vi "Oxford-1820-Main.vi"() -> ()   [LabVIEW 2016]
uses:
  <instrlib>/Mercury iXX/Public/Controls/Unit String.ctl
  <instrlib>/Mercury iXX/Public/Libraries/Heater/Controls/Heater Device (Read).ctl
  <instrlib>/Mercury iXX/Public/Controls/Manufacturing Data.ctl
  <instrlib>/Mercury iXX/Public/Libraries/Heater/Controls/Heater Signals Cluster.ctl
  <instrlib>/Mercury iXX/Public/Libraries/Level Meter/Controls/Level Meter (Read).ctl
  <instrlib>/Mercury iXX/Public/Libraries/Level Meter/Controls/Nitrogen Configuration.ctl
  <instrlib>/Mercury iXX/Public/Libraries/Level Meter/Controls/Frequency Configuration.ctl
  <instrlib>/Mercury iXX/Public/Libraries/Level Meter/Controls/Signals.ctl
  <instrlib>/Mercury iXX/Public/Libraries/Level Meter/Controls/Helium Configuration.ctl
  <instrlib>/Mercury iXX/Public/Libraries/Level Meter/Controls/Resistance Configuration.ctl
  <instrlib>/Mercury iXX/Public/Libraries/Level Meter/Controls/Pre-Pulse.ctl
  <instrlib>/Mercury iXX/Public/Libraries/Level Meter/Controls/Pulse.ctl
  <instrlib>/Mercury iXX/Public/Libraries/Auxiliary/Controls/AUX Device (Read).ctl
  <instrlib>/Mercury iXX/Public/Libraries/Auxiliary/Controls/AUX Signals (Read).ctl
  <instrlib>/Mercury iXX/Public/Libraries/Magnet/Controls/Device (Read).ctl
  <instrlib>/Mercury iXX/Public/Libraries/Magnet/Controls/Signals (Read).ctl
  <instrlib>/Mercury iXX/Public/Libraries/Magnet/Controls/Identifier.ctl
  <instrlib>/Mercury iXX/Public/Libraries/Temperature/Controls/Calibration Cluster.ctl
  <instrlib>/Mercury iXX/Public/Libraries/Temperature/Controls/Calibration Interpolation.ctl
  <instrlib>/Mercury iXX/Public/Libraries/Temperature/Controls/Excitation Cluster.ctl
  <instrlib>/Mercury iXX/Public/Libraries/Temperature/Controls/Excitation Type.ctl
  <instrlib>/Mercury iXX/Public/Libraries/Pressure/Controls/Pressure Signals Cluster.ctl
  <instrlib>/Mercury iXX/Public/Controls/Mercury Reference.ctl
  <instrlib>/Mercury iXX/Public/Controls/Comms Transport Layer.ctl
  <instrlib>/Mercury iXX/Private/Controls/Query Dynamic Reference.ctl
  Mercury - Typedefs/Status.ctl
  <instrlib>/Mercury iXX/Public/Libraries/Magnet/Controls/PSU Actions.ctl
  Mercury - Typedefs/Actions.ctl
  <instrlib>/Mercury iXX/Public/Libraries/Magnet/Controls/Switch Heater.ctl
  <instrlib>/Mercury iXX/Public/Controls/ISOBus Address.ctl
  <instrlib>/Mercury iXX/Public/Controls/Response String.ctl
  <userlib>/_OpenG.lib/error/error.llb/Filter Error Codes (Array)__ogtk.vi
  <instrlib>/Mercury iXX/Public/Libraries/System/Open/Open System.vi
  <instrlib>/Mercury iXX/Public/Libraries/System/Read/Catalogue (Read).vi
  <instrlib>/Mercury iXX/Public/Libraries/System/Read/Display Automatic Dimming (Read).vi
  <instrlib>/Mercury iXX/Public/Libraries/System/Read/Display Automatic Dimming Time (Read).vi
  <instrlib>/Mercury iXX/Public/Libraries/System/Read/Display Brightness (Read).vi
  <instrlib>/Mercury iXX/Public/Libraries/System/Read/Date (Read).vi
  <instrlib>/Mercury iXX/Public/Libraries/System/Read/Time (Read).vi
  <instrlib>/Mercury iXX/Public/Libraries/System/Read/DateTime (Read).vi
  <instrlib>/Mercury iXX/Public/Libraries/System/Read/HVer (Read).vi
  <instrlib>/Mercury iXX/Public/Libraries/System/Read/FVer (Read).vi
  <instrlib>/Mercury iXX/Public/Libraries/System/Read/Serial Number (Read).vi
  <instrlib>/Mercury iXX/Public/Libraries/System/Read/Flash Space (Read).vi
  <instrlib>/Mercury iXX/Public/Libraries/System/Read/Mode (Read).vi
  <instrlib>/Mercury iXX/Public/Libraries/System/Set/DateTime (Set).vi
  <instrlib>/Mercury iXX/Public/Libraries/Temperature/Open/Open Temperature Device.vi
  <instrlib>/Mercury iXX/Public/Libraries/Temperature/Configuration/Read/Serial Number (Read).vi
  <instrlib>/Mercury iXX/Public/Libraries/Temperature/Configuration/Read/Nickname (Read).vi
  <instrlib>/Mercury iXX/Public/Libraries/Temperature/Configuration/Read/Excitation Magnitude (Read).vi
  <instrlib>/Mercury iXX/Public/Libraries/Temperature/Configuration/Read/Temperature Sensor (Read).vi
  <instrlib>/Mercury iXX/Public/Libraries/Temperature/Configuration/Read/Excitation Type (Read).vi
  <instrlib>/Mercury iXX/Public/Libraries/Temperature/Configuration/Read/Calibration Hot Limit (Read).vi
  <instrlib>/Mercury iXX/Public/Libraries/Temperature/Configuration/Read/Calibration Cold Limit (Read).vi
  <instrlib>/Mercury iXX/Public/Libraries/Temperature/Signals/Read/Voltage (Read).vi
  <instrlib>/Mercury iXX/Public/Libraries/Temperature/Signals/Read/Temperature (Read).vi
  <instrlib>/Mercury iXX/Public/Libraries/Temperature/Configuration/Read/Temperature Device (Read).vi
  <instrlib>/Mercury iXX/Public/Libraries/Heater/Open/Open Heater Device.vi
  <instrlib>/Mercury iXX/Public/Libraries/Heater/Configuration/Read/Heater Device (Read).vi
  <instrlib>/Mercury iXX/Public/Libraries/Heater/Configuration/Read/Nickname (Read).vi
  <instrlib>/Mercury iXX/Public/Libraries/Heater/Configuration/Read/Serial Number (Read).vi
  <instrlib>/Mercury iXX/Public/Libraries/Heater/Configuration/Read/Voltage Limit (Read).vi
  <instrlib>/Mercury iXX/Public/Libraries/Heater/Configuration/Read/Nominal Resistance (Read).vi
  <instrlib>/Mercury iXX/Public/Libraries/Heater/Configuration/Read/Maximum Power (Read).vi
  <instrlib>/Mercury iXX/Public/Libraries/Heater/Signals/Read/Voltage (Read).vi
  <instrlib>/Mercury iXX/Public/Libraries/Heater/Signals/Read/Power (Read).vi
  <instrlib>/Mercury iXX/Public/Libraries/Heater/Signals/Read/Current (Read).vi
  <instrlib>/Mercury iXX/Public/Libraries/Auxiliary/Open/Open Auxiliary Device.vi
  <instrlib>/Mercury iXX/Public/Libraries/Auxiliary/Configuration/Read/Aux Device (Read).vi
  <instrlib>/Mercury iXX/Public/Libraries/Auxiliary/Configuration/Read/Serial Number (Read).vi
  <instrlib>/Mercury iXX/Public/Libraries/Auxiliary/Configuration/Read/Minimum Gas Flow (Read).vi
  <instrlib>/Mercury iXX/Public/Libraries/Auxiliary/Configuration/Read/Gas Flow Scaling (Read).vi
  <instrlib>/Mercury iXX/Public/Libraries/Auxiliary/Configuration/Read/Temperature Error Sensitivity (Read).vi
  <instrlib>/Mercury iXX/Public/Libraries/Auxiliary/Configuration/Read/Temperature Error Voltage Sensitivity (Read).vi
  <instrlib>/Mercury iXX/Public/Libraries/Auxiliary/Configuration/Read/Valve Gearing (Read).vi
  <instrlib>/Mercury iXX/Public/Libraries/Auxiliary/Configuration/Read/Stepper Speed (Read).vi
  <instrlib>/Mercury iXX/Public/Libraries/Auxiliary/Signals/Read/Position (Read).vi
  <instrlib>/Mercury iXX/Public/Libraries/Auxiliary/Signals/Read/Percent Open (Read).vi
  <instrlib>/Mercury iXX/Public/Libraries/Pressure/Open/Open Pressure Device.vi
  <instrlib>/Mercury iXX/Public/Libraries/Pressure/Configuration/Read/Pressure Device (Read).vi
  <instrlib>/Mercury iXX/Public/Libraries/Pressure/Configuration/Read/Nickname (Read).vi
  <instrlib>/Mercury iXX/Public/Libraries/Pressure/Signals/Read/Current (Read).vi
  <instrlib>/Mercury iXX/Public/Libraries/Pressure/Signals/Read/Voltage (Read).vi
  <instrlib>/Mercury iXX/Public/Libraries/Level Meter/Open/Open Level Meter Device.vi
  <instrlib>/Mercury iXX/Public/Libraries/Level Meter/Configuration/Read/Level Meter Device (Read).vi
  <instrlib>/Mercury iXX/Public/Libraries/Level Meter/Configuration/Read/Serial Number (Read).vi
  <instrlib>/Mercury iXX/Public/Libraries/Level Meter/Configuration/Read/Helium Probe Resistance (Read).vi
  <instrlib>/Mercury iXX/Public/Libraries/Level Meter/Configuration/Read/Helium Pulse Mag (Read).vi
  <instrlib>/Mercury iXX/Public/Libraries/Level Meter/Configuration/Read/Helium Pulse Duration (Read).vi
  <instrlib>/Mercury iXX/Public/Libraries/Level Meter/Configuration/Read/Nitrogen Freq at 100 (Read).vi
  <instrlib>/Mercury iXX/Public/Libraries/Level Meter/Configuration/Read/Nitrogen Pulse Count Period (Read).vi
  <instrlib>/Mercury iXX/Public/Libraries/Level Meter/Signals/Read/Probe Resistance Helium (Read).vi
  <instrlib>/Mercury iXX/Public/Libraries/Level Meter/Signals/Read/Probe Level Helium (Read).vi
  <instrlib>/Mercury iXX/Public/Libraries/Level Meter/Signals/Read/Probe Count Nitrogen (Read).vi
  <instrlib>/Mercury iXX/Public/Libraries/Level Meter/Signals/Read/Probe Level Nitrogen (Read).vi
  <instrlib>/Mercury iXX/Public/Libraries/Magnet/Open/Open Magnet Device.vi
  <instrlib>/Mercury iXX/Public/Libraries/Magnet/Configuration/Read/Magnet Device (Read).vi
  <instrlib>/Mercury iXX/Public/Libraries/Magnet/Configuration/Read/Serial Number (Read).vi
  <instrlib>/Mercury iXX/Public/Libraries/Magnet/Configuration/Read/Bipolar Output (Read).vi
  <instrlib>/Mercury iXX/Public/Libraries/Magnet/Configuration/Read/Output Configuration (Read).vi
  <instrlib>/Mercury iXX/Public/Libraries/Magnet/Configuration/Read/Current Limit (Read).vi
  <instrlib>/Mercury iXX/Public/Libraries/Magnet/Configuration/Read/Current to Field Factor (Read).vi
  <instrlib>/Mercury iXX/Public/Libraries/Magnet/Configuration/Read/Switch Present (Read).vi
  <instrlib>/Mercury iXX/Public/Libraries/Magnet/Configuration/Read/Software Voltage Limit (Read).vi
  <instrlib>/Mercury iXX/Public/Libraries/Magnet/Signals/Read/Current Rate (Read).vi
  <instrlib>/Mercury iXX/Public/Libraries/Magnet/Configuration/Read/PSU Action Status (Read).vi
  <instrlib>/Mercury iXX/Public/Libraries/Temperature/Signals/Read/Resistance (Read).vi
  <instrlib>/Mercury iXX/Public/Libraries/Temperature/Configuration/Set/Excitation Magnitude (Set).vi
  <instrlib>/Mercury iXX/Public/Libraries/Magnet/Signals/Read/Switch Heater Status (Read).vi
  <instrlib>/Mercury iXX/Public/Libraries/Magnet/Signals/Read/Current (Read).vi
  <instrlib>/Mercury iXX/Public/Libraries/Magnet/Signals/Read/Voltage (Read).vi
  <instrlib>/Mercury iXX/Public/Libraries/Magnet/Signals/Read/Field (Read).vi
  <instrlib>/Mercury iXX/Public/Libraries/Magnet/Signals/Read/Target Field Rate (Read).vi
  <instrlib>/Mercury iXX/Public/Libraries/Magnet/Signals/Read/Target Field (Read).vi
  <instrlib>/Mercury iXX/Public/Libraries/Magnet/Signals/Read/Persistant Field (Read).vi
  <instrlib>/Mercury iXX/Public/Libraries/Magnet/Configuration/Set/PSU Action Status (Set).vi
  <instrlib>/Mercury iXX/Public/Libraries/Magnet/Signals/Read/Persistant Current (Read).vi
  <instrlib>/Mercury iXX/Public/Libraries/Magnet/Signals/Set/Switch Heater No Check (Set).vi
  <instrlib>/Mercury iXX/Public/Libraries/Magnet/Signals/Set/Target Field Rate (Set).vi
  <instrlib>/Mercury iXX/Public/Libraries/Magnet/Signals/Set/Target Field (Set).vi
  <instrlib>/Mercury iXX/Public/Libraries/Lambda/Open/Open Lambda Device.vi
  <instrlib>/Mercury iXX/Public/Libraries/Lambda/Configuration/Set/Lambda Flow Auto (Set).vi
  <instrlib>/Mercury iXX/Public/Libraries/Level Meter/Configuration/Set/Pulse Slow-Fast (Set).vi
  <instrlib>/Mercury iXX/Public/Libraries/Lambda/Configuration/Set/Lambda Percentage Flow (Set).vi
  <instrlib>/Mercury iXX/Mercury iXX.lvlib
  <instrlib>/Mercury iXX/Public/Libraries/Pressure.lvlib
  <instrlib>/Mercury iXX/Public/Libraries/System.lvlib
  <instrlib>/Mercury iXX/Public/Libraries/Temperature.lvlib
  <instrlib>/Mercury iXX/Public/Libraries/Auxiliary.lvlib
  <instrlib>/Mercury iXX/Public/Libraries/Magnet.lvlib
  <instrlib>/Mercury iXX/Public/Libraries/Level Meter.lvlib
  <instrlib>/Mercury iXX/Public/Libraries/Lambda.lvlib
  <instrlib>/Mercury iXX/Public/Libraries/System/Controls/User Mode.ctl
  <instrlib>/Mercury iXX/Public/Libraries/System/Set/Mode (Set).vi
  <instrlib>/Mercury iXX/Public/Libraries/Heater.lvlib
  <instrlib>/Mercury iXX/Public/Libraries/Magnet/Configuration/Set/Switch Heater Current (Set).vi
panel:
  out "LPF ON":timestamp
  in  "Tab Control":T1(tab)
  out "LEDs":bool[](array[boolean])
  out "Iteration Time":dbl
  in  "Percentage Open":dbl=100.0 format="%#_13g"
  out "PS Heat on or off (sec)":dbl format="%<%H:%M:%S>t"
  out "LPF on (min)":dbl=5373.0 format="%<%H:%M:%S>t"
  out "Magnet Status 2":string
  in  "OK":bool
  out "LPF Resistance":dbl=4.2075 format="%_3f ohms"
  out "Magnet Resistance":dbl=3.8705 format="%_3f ohms"
  out "ETA":timestamp format="%<%I:%M:%S %p\n%m/%d/%y>T"
  in  "Open Needle Valve":bool
  in  "Close Needle Valve":bool
  in  "Lambda":bool
  out "LPF Pressure":dbl format="%_5f mB"
  out "LPF Needle Valve (%)":dbl format="%_6g"
  out "LPF Temperature":dbl=4.2075 format="%_2f K"
  out "Magnet Temperature":dbl=3.8705 format="%_2f K"
  out "He LVL Chart":dbl(slide)=52.0833 scale=0.0..100.0
  out "N2 LVL Chart":dbl(slide)=61.3025 scale=0.0..100.0
  in  "Remote Mode":bool
  out "Power Supply Field (T)":dbl=0.0001 format="%#.5f"
  out "Magnet Field (T)":dbl format="%.5f"
  out "Voltage (V)":dbl=-0.0003 format="%.5f"
  out "Current (A)":dbl=0.0006 format="%.5f"
  out "N2 LEVEL":dbl=61.3025 format="%.0f %"
  out "He LEVEL":dbl=52.0833 format="%.0f %"
  in  "Fast/Slow Fill":bool
  out "Magnet Field (T)":dbl(knob) caption="Voltage (V)" scale=-20.0..20.0
  out "SWITCH HEATER":bool
  in  "PS Heat":bool
  in  "Clamp":bool
  in  "To Set":bool
  in  "To Zero":bool
  in  "Hold":bool
  out "Magnet Status":string="Clamped"
  out "Target Field Rate (T/min)":dbl=1.0 format="%.5f"
  out "Target Field (T)":dbl format="%#.5f"
  in  "Target Rate (T/min)":dbl=0.1 format="%.5f"
  in  "Target Field (T)":dbl format="%#.5f"
  in  "Send to IPS":bool
  out "Voltage (V)":dbl(knob)=-0.0003 scale=-10.0..10.0
  out "Current (A)":dbl(knob)=0.0006 scale=-180.0..180.0
  in  "Mercury Functions":T2(tab)=enum."ITC: Temperature"
  out "time stamp":timestamp=timestamp(3543841780 s since 1904-01-01)
  out "Free Space":i32=166384 caption="Free Space (KB)"
  out "Set Date Response":string="VALID"
  out "String":string="NORM" caption="User Mode"
  out "Date":string="2016:04:18"
  out "Time":string="11:29:40"
  out "Hardware Version":string="65"
  out "Firmware Version":string="2.2.6.20"
  out "Serial Number":string="154650110"
  out "ITC Devices":string[](array[string])=["DB4.G1:AUX", "DB8.P1:PRES", "MB0.H1:HTR", "MB1.T1:TEMP"]
  out "S/W Version(s)":string[](array[string])=["2.2.6.20\n"]
  out "Serial Number(s)":string[](array[string])=["154650110"]
  out "# of Instruments":i32=1
  out "Automatic Dimming":string="OFF"
  out "Dimming Time":string="5"
  out "Display Brightness":string="100"
  in  "ITC IP Address":string="130.49.180.101"
  out "Excitation Magnitude":dbl=5.0
  out "Sensor Type":string="NTC"
  out "Excitation Type":string="UNIP"
  out "Hot Limit":dbl=1000.0
  out "H Unit":T3="K"
  out "Cold Limit":dbl=1000.0
  out "C Unit":T3="K"
  out "Unit":T3
  out "Voltage":dbl=0.005
  out "V Unit":T3="V"
  out "Temperature":dbl=4.2075
  out "T Unit":T3="K"
  out "Temp S/N":string="154650110"
  out "T Nickname":string="Mag_AB_MB1"
  out "ITC Calibration":T4
  out "ITC Excitation":T6
  out "ITC Manufacturing":T8
  out "Heater Device Settings":T9={"Manufacturing"={"Hardware Version"="65", "Firmware Version"="2.3", "Serial Number"="154650110"}, "Nickname"="MB0.H1", "Voltage Limit"="1", "Nominal Resistance"="10", "Maximum Power"="0.1000", "Heater Signals"={"Voltage"="0.0507V", "Current"="-0.0000A", "Power"="0.0000W"}, "Status"="2"}
  out "Htr C Unit":T3="A"
  out "Htr P Unit":T3="W"
  out "Htr V Unit":T3="V"
  out "Htr Current":dbl=-0.0
  out "Htr Power":dbl
  out "Htr Voltage":dbl=0.0507
  out "Power Unit":T3
  out "Volt Unit":T3
  out "Res Unit":T3
  out "Maximum Power":dbl=0.1
  out "Htr Resistance":dbl=10.0
  out "Htr Voltage Limit":dbl=1.0
  out "Htr S/N":string="154650110"
  out "Htr Nickname":string="MB0.H1"
  out "Nickname":string="Lam_P_DB8"
  out "Current":dbl=-0.0
  out "Voltage":dbl=-8.219999999999999e-05
  out "Manufacturing":T8
  out "Pressure Signals":T11
  out "Auxiliary Device Details":T12={"Manufacturing"={"Hardware Version"="65", "Firmware Version"="3.1", "Serial Number"="154650084"}, "Min Flow"=0.0, "Scaling Factor"=50.0, "Temp Err"=9.0, "Temp V Err"=11.0, "Gear"=2, "Speed"=2, "Signals"={"Position"=0.0, "% Open"=0.0, "I0"="ON", "I1"="OFF", "I2"="OFF", "I3"="OFF", "O0"="OFF", "O1"="OFF", "O2"="OFF", "O3"="OFF"}, "Nickname"="DB4.G1", "Status"="0"} {"Signals"."% Open" min=0.0 max=100.0 step=0.1 format="%.4f"; "Signals"."Position" max=20.0 step=1.0 format="%.4f"; "Speed" max=7 step=1; "Gear" max=7 step=1; "Temp V Err" min=0.0 max=20.0 step=0.1; "Temp Err" min=0.0 max=20.0 step=0.1; "Scaling Factor" min=0.0 max=99.0 step=0.1; "Min Flow" min=0.0 max=20.0 step=0.1}
  out "Aux S/N":string="154650084"
  out "Min Flow":dbl caption="Minimum Gas Flow" format="%#.1f"
  out "Scaling Factor":dbl=50.0 caption="Gas Flow Scaling Factor" format="%#.1f"
  out "Temp Err":dbl=9.0 caption="Temperature Error Sensitivity" format="%#.1f"
  out "Temp V Err":dbl=11.0 caption="Temperature Voltage Error Sensitivity" format="%#.1f"
  out "Gear":u32=2 caption="Valve Gearing"
  out "Speed":u32=2 caption="Stepper Speed"
  out "Unit 2":T3
  out "Unit 3":T3
  out "Unit 4":T3
  out "Unit 5":T3
  out "Unit 6":T3
  out "Unit 7":T3
  out "Position":u32
  out "% Open":dbl caption="Percentage Open (%)"
  out "Unit":T3
  out "Unit":T3="%"
  out "time stamp 2":timestamp=timestamp(3543841781 s since 1904-01-01)
  out "Free Space 2":i32=166316 caption="Free Space (KB)"
  out "Set Date Response 2":string="VALID"
  out "String 2":string="NORM" caption="User Mode"
  out "Date 2":string="2016:04:18"
  out "Time 2":string="11:29:45"
  out "Hardware Version 2":string="65"
  out "Firmware Version 2":string="2.2.6.20"
  out "Serial Number 2":string="153350063"
  out "IPS Devices":string[](array[string])=["DB3.L1:LVL", "GRPX:PSU", "GRPY:PSU", "GRPZ:PSU", "MB1.T1:TEMP", "PSU.M1:PSU", "PSU.M2:PSU", "PSU.M3:PSU"]
  out "S/W Version(s) 2":string[](array[string])=["2.2.6.20\n"]
  out "Serial Number(s) 2":string[](array[string])=["153350063"]
  out "# of Instruments 2":i32=1
  out "Automatic Dimming 2":string="OFF"
  out "Dimming Time 2":string="5"
  out "Display Brightness 2":string="100"
  in  "IPS IP Address":string="130.49.180.102"
  out "LVL Device DetailSettings":T14={"Manufacturing"={"Hardware Version"="65", "Firmware Version"="2.2", "Serial Number"="152450013"}, "Nitrogen Configuration"={"Frequency Configuration"={"Freq 0%"=0.0, "Freq 100%"=0.0}, "Pulse Period"=0.0}, "Signals"={"Helium Signals"={"Resistance"=75.5626, "Level"=52.0833}, "Nitrogen Signals"={"Count"=8800.0, "Freq"=487361.0, "Level"=61.3445}}, "Nickname"="DB3.L1", "Status"="0", "Helium Configuration"={"Resistance Configuration"={"Res 0%"=0.0, "Res 100%"=0.0}, "Pre-Pulse"={"Magnitude"=0.0, "Duration"=0.0}, "Pulse"={"Magnitude"=0.0, "Duration"=0.0, "Delay"=0.0}}}
  out "LVL S/N":string="152450013"
  out "LVL P Magnitude":dbl=125.0 caption="Pulse Magnitude (mA)"
  out "LVL P Duration":dbl=5.0 caption="Pulse Duration (s)"
  out "N Freq 100%":dbl=7880.0 caption="Frequency at 100% (Hz)"
  out "N Pulse Period":dbl=1000.0 caption="Pulse Period (ms)"
  out "He Res Config":T19={"Res 0%"=149.0, "Res 100%"=8.0}
  out "He Resistance":dbl=75.5626 caption="Resistance (Ohms)"
  out "He Level":dbl=52.0833 caption="Helium Level (%)"
  out "N Counter":u32 caption="Counter"
  out "N Level":dbl=61.3445 caption="Nitrogen Level (%)"
  out "Excitation Magnitude 2":dbl=5.0
  out "Sensor Type 2":string="NTC"
  out "Excitation Type 2":string="UNIP"
  out "Hot Limit 2":dbl=1000.0
  out "H Unit 2":T3="K"
  out "Cold Limit 2":dbl=1000.0
  out "C Unit 2":T3="K"
  out "Unit 12":T3
  out "Voltage 2":dbl=0.005
  out "V Unit 2":T3="V"
  out "Temperature 2":dbl=3.8706
  out "T Unit 2":T3="K"
  out "Temp S/N 2":string="153350063"
  out "T Nickname 2":string="MB1.T1"
  out "IPS Calibration":T4
  out "IPS Excitation":T6
  out "IPS Manufacturing":T8
  out "Magnet Device Details":T22={"Manufacturing"={"Hardware Version"="NOT_FOUND", "Firmware Version"="NOT_FOUND", "Serial Number"="NOT_FOUND"}, "Nickname"="GRPZ", "Bipolar Output"="ON", "String"="PARA", "Current Limit"=174.0, "AtoB"=8.688, "Inductance"=39.406, "Switch Present"="PSU.M1", "Swh Htr Current"=86.0, "SW VLIM"=9.0, "V Trans Time"=1000.0, "Magnet PSU Signals"={"Voltage"=-0.0002, "Current"=0.0002, "Current Rate"=100.0, "Field"=0.0001, "Field Rate"=11.5101, "Persistant Current"=0.0003, "Persistant Field"=0.0, "Target Current"=0.0, "Target Field"=0.0, "Target Current Rate"=8.688, "Target Field Rate"=1.0, "Switch Heater Status (SWHT)"="OFF", "Switch Heater Status (SWHN)"="OFF"}, "PSU Action"="CLMP", "Status"="40000000", "Level Limit"=0.0, "Temperature Limit"=999.0} {"Temperature Limit" format="%#.1f"; "Level Limit" format="%#.1f"; "V Trans Time" format="%#.1f"; "SW VLIM" format="%#.1f"; "Swh Htr Current" format="%#.1f"; "Inductance" format="%#.1f"; "AtoB" format="%#.1f"; "Current Limit" format="%#.1f"}
  out "Mag S/N":string="NOT_FOUND"
  out "Bipolar Output":string="ON"
  out "Out Config":string="PARA" caption="Output Configuration"
  out "Current Limit":dbl=174.0 caption="Current Limit (A)" format="%#.1f"
  out "AtoB":dbl=8.688 caption="Current Field Factor (A/T)" format="%#.1f"
  out "Switch Present":string="PSU.M1"
  out "SW VLIM":dbl=9.0 caption="Software Voltage Limit (V)" format="%#.1f"
  out "Unit 8":T3
  out "Unit 9":T3
  out "Unit 10":T3
  out "Current Rate":dbl=100.0
  out "PSU Act Stat":string="CLMP" caption="PSU Action Status"
  out "Unit 11":T3="A/min"
  in  "Device Identifier":T24="GRPZ"
  out "M3 Voltage":dbl
  out "M3 Current":dbl
  out "M2 Voltage":dbl
  out "M2 Current":dbl
  out "M1 Voltage":dbl
  out "M1 Current":dbl
  out "Error List":T25(array[cluster])
  out "PS ON/OFF":timestamp format="%<%I:%M:%S %p>T"
  # "v2017/09/27"
  # "Voltage (V)"
  # "Magnet (T)"
  # "Current (A)"
  # "Slow Rates\nCurrent Range (A)     Field Range (T)    Rate (T/min)\n0       -- 100        0    -- 11.5       0.91\n100     -- 150        11.5 -- 17.2       0.23\n150     -- 155.467    17.2 -- 18         0.11\n155.567 -- 172.471    18   -- 20         0.11"
  # "Fast Rates\nCurrent Range (A)     Field Range (T)    Rate (T/min)\n0       -- 155.467    0    -- 18         1.0\n155.567 -- 172.471    18   -- 20         0.25"
  # "ITC: 101\nIPS: 102\nIPS VR: 67"
  # "ITC: 101\nIPS: 102\nIPS VR: 67"
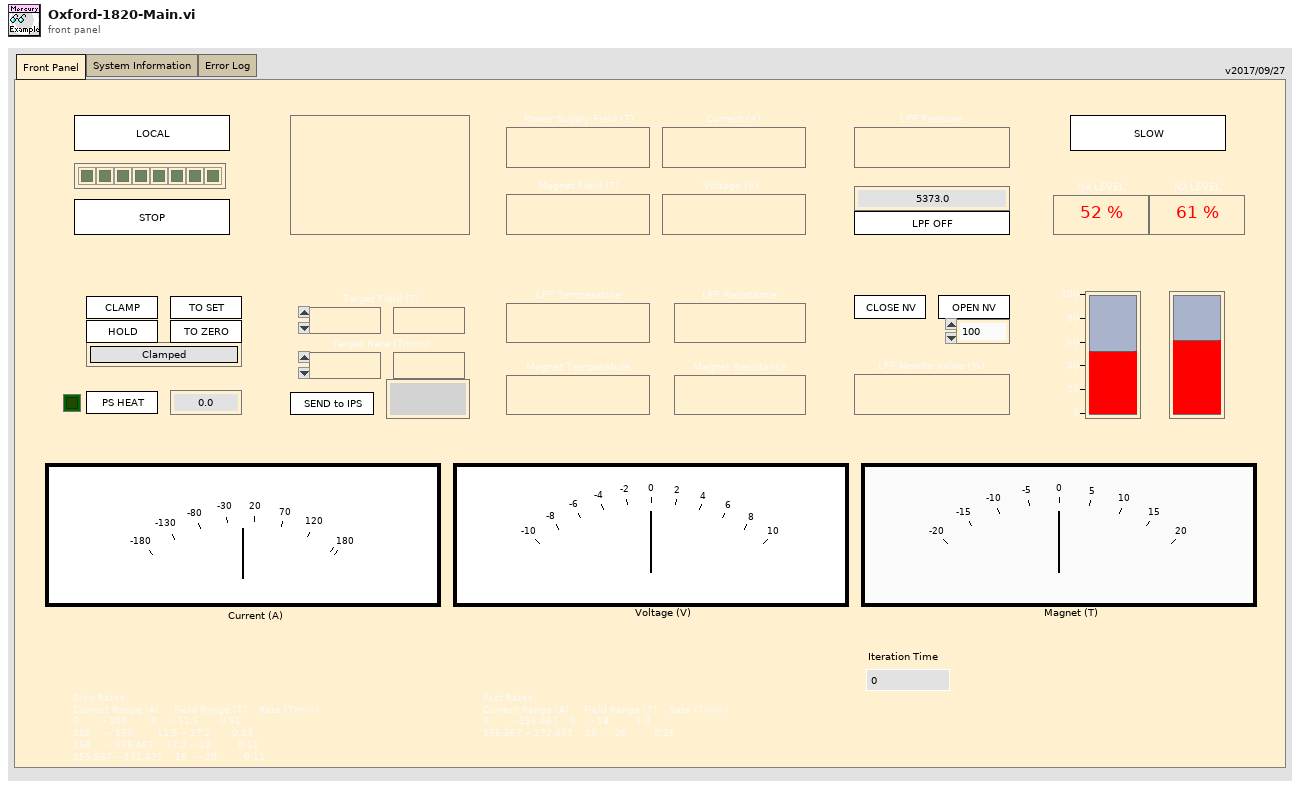
[diagram p1: front panel]
types:
  T1 = enum32{"Front Panel", "System Information", "Error Log"}
  T2 = enum32{"ITC: System", "ITC: Temperature", "ITC: Heater", "ITC: Pressure", "ITC: Auxiliary", "IPS: System", "IPS: Level Meter", "IPS: Temperature", "IPS: Magnet"}
  T3 = typedef "Mercury iXX.lvlib/Unit String.ctl" = string
  T4 = typedef "Mercury iXX.lvlib/Temperature.lvlib/Calibration Cluster.ctl" = cluster{"Filename":string, "Interpolation":T5, "Scaling Factor":string, "Offset Factor":string, "Hot Limit":string, "Cold Limit":string, "Last Calibration":string, "Reference":string}
  T5 = typedef "Mercury iXX.lvlib/Temperature.lvlib/Calibration Interpolation.ctl" = string
  T6 = typedef "Mercury iXX.lvlib/Temperature.lvlib/Excitation Cluster.ctl" = cluster{"Excitation Type":T7, "Magnitude":string}
  T7 = typedef "Mercury iXX.lvlib/Temperature.lvlib/Excitation Type.ctl" = string
  T8 = typedef "Mercury iXX.lvlib/Manufacturing Data.ctl" = cluster{"Hardware Version":string, "Firmware Version":string, "Serial Number":string}
  T9 = typedef "Mercury iXX.lvlib/Heater.lvlib/Heater Device (Read).ctl" = cluster{"Manufacturing":T8, "Nickname":string, "Voltage Limit":string, "Nominal Resistance":string, "Maximum Power":string, "Heater Signals":T10, "Status":string}
  T10 = typedef "Mercury iXX.lvlib/Heater.lvlib/Heater Signals Cluster.ctl" = cluster{"Voltage":string, "Current":string, "Power":string}
  T11 = typedef "Mercury iXX.lvlib/Pressure.lvlib/Pressure Signals Cluster.ctl" = cluster{"Voltage":string, "Current":string, "Power":string, "Pressure":string}
  T12 = typedef "Mercury iXX.lvlib/Auxiliary.lvlib/AUX Device (Read).ctl" = cluster{"Manufacturing":T8, "Min Flow":dbl, "Scaling Factor":dbl, "Temp Err":dbl, "Temp V Err":dbl, "Gear":u32, "Speed":u32, "Signals":T13, "Nickname":string, "Status":string}
  T13 = typedef "Mercury iXX.lvlib/Auxiliary.lvlib/AUX Signals (Read).ctl" = cluster{"Position":dbl, "% Open":dbl, "I0":string, "I1":string, "I2":string, "I3":string, "O0":string, "O1":string, "O2":string, "O3":string}
  T14 = typedef "Mercury iXX.lvlib/Level Meter.lvlib/Level Meter (Read).ctl" = cluster{"Manufacturing":T8, "Nitrogen Configuration":T15, "Signals":T17, "Nickname":string, "Status":string, "Helium Configuration":T18}
  T15 = typedef "Mercury iXX.lvlib/Level Meter.lvlib/Nitrogen Configuration.ctl" = cluster{"Frequency Configuration":T16, "Pulse Period":dbl}
  T16 = typedef "Mercury iXX.lvlib/Level Meter.lvlib/Frequency Configuration.ctl" = cluster{"Freq 0%":dbl, "Freq 100%":dbl}
  T17 = typedef "Mercury iXX.lvlib/Level Meter.lvlib/Signals.ctl" = cluster{"Helium Signals":cluster{"Resistance":dbl, "Level":dbl}, "Nitrogen Signals":cluster{"Count":dbl, "Freq":dbl, "Level":dbl}}
  T18 = typedef "Mercury iXX.lvlib/Level Meter.lvlib/Helium Configuration.ctl" = cluster{"Resistance Configuration":T19, "Pre-Pulse":T20, "Pulse":T21}
  T19 = typedef "Mercury iXX.lvlib/Level Meter.lvlib/Resistance Configuration.ctl" = cluster{"Res 0%":dbl, "Res 100%":dbl}
  T20 = typedef "Mercury iXX.lvlib/Level Meter.lvlib/Pre-Pulse.ctl" = cluster{"Magnitude":dbl, "Duration":dbl}
  T21 = typedef "Mercury iXX.lvlib/Level Meter.lvlib/Pulse.ctl" = cluster{"Magnitude":dbl, "Duration":dbl, "Delay":dbl}
  T22 = typedef "Mercury iXX.lvlib/Magnet.lvlib/Device (Read).ctl" = cluster{"Manufacturing":T8, "Nickname":string, "Bipolar Output":string, "String":string, "Current Limit":dbl, "AtoB":dbl, "Inductance":dbl, "Switch Present":string, "Swh Htr Current":dbl, "SW VLIM":dbl, "V Trans Time":dbl, "Magnet PSU Signals":T23, "PSU Action":string, "Status":string, "Level Limit":dbl, "Temperature Limit":dbl}
  T23 = typedef "Mercury iXX.lvlib/Magnet.lvlib/Signals (Read).ctl" = cluster{"Voltage":dbl, "Current":dbl, "Current Rate":dbl, "Field":dbl, "Field Rate":dbl, "Persistant Current":dbl, "Persistant Field":dbl, "Target Current":dbl, "Target Field":dbl, "Target Current Rate":dbl, "Target Field Rate":dbl, "Switch Heater Status (SWHT)":string, "Switch Heater Status (SWHN)":string}
  T24 = typedef "Mercury iXX.lvlib/Magnet.lvlib/Identifier.ctl" = string
  T25 = cluster{"time":timestamp, "code":i32, "source":string}[]
  T26 = enum32{"invalid app kind", "Development System", "Run Time System", "Student Edition", "Embedded LabVIEW", "Evaluation", "Custom"}
  T27 = cluster{"time":timestamp, "code":i32, "source":string}
  T28 = enum32{"Invalid", "Standard", "Closed", "Hidden", "Minimized", "Maximized"}
  T29 = typedef "Status.ctl" = cluster{"Magnet Field":dbl, "PS Field":dbl, "Target Field":dbl, "Target Field Rate":dbl, "Voltage":dbl, "Current":dbl, "Switch":bool, "Mercury State":string}
  T30 = cluster{"Magnet Field":dbl, "PS Field":dbl, "Target Field":dbl, "Target Field Rate":dbl, "Voltage":dbl, "Current":dbl}
  T31 = typedef "Actions.ctl" = cluster{"Hold":bool, "Clamp":bool, "To Set":bool, "To Zero":bool, "Send to IPS":bool, "PS Heat":bool, "Lambda":bool}
  T32 = typedef "Mercury iXX.lvlib/Magnet.lvlib/PSU Actions.ctl" = string
  T33 = typedef "Mercury iXX.lvlib/Magnet.lvlib/Switch Heater.ctl" = string
  T34 = typedef "Mercury iXX.lvlib/ISOBus Address.ctl" = i32
  T35 = typedef "Mercury iXX.lvlib/Response String.ctl" = string
  T36 = typedef "Mercury iXX.lvlib/Mercury Reference.ctl" = cluster{"Comms":refnum<visa-resource-name>, "Device ID":string[], "Comms Layer":T37, "Command":string, "Query reference":T38}
  T37 = typedef "Mercury iXX.lvlib/Comms Transport Layer.ctl" = enum16{"Ethernet TCP/IP", "USB", "ISOBus - RS-232", "GPIB"}
  T38 = typedef "Mercury iXX.lvlib/Query Dynamic Reference.ctl" = refnum<vi>
  T39 = cluster{"Core":cluster{"Current VI Reference":refnum<vi>, "Close Panel on Exit?":bool}, "Mercury ITC Ref":T36, "Mercury IPS Ref":T36, "sentinel":bool, "Error Log":cluster{"time":timestamp, "code":i32, "source":string}[], "read ITC T?":bool, "counter":i32}
  T40 = typedef "Filtered Error Details - Cluster__ogtk.ctl" = cluster{"code":i32, "source":string}
  T41 = cluster{"Current VI Reference":refnum<vi>, "Close Panel on Exit?":bool}
  T42 = typedef "Mercury iXX.lvlib/System.lvlib/User Mode.ctl" = string
  T43 = typedef "Mercury iXX.lvlib/Temperature.lvlib/Temperature Sensor Type.ctl" = string
  T44 = typedef "Mercury iXX.lvlib/Temperature.lvlib/Temperature Device (Read).ctl" = cluster{"Manufacturing":T8, "Temperature Sensor Type":T43, "Excitation":T6, "Calibration":T4, "Control Loop":T45, "Temperature Signals":T46, "Nickname":string, "Status":string}
  T45 = typedef "Mercury iXX.lvlib/Temperature.lvlib/Loop Cluster.ctl" = cluster{"Heater":string, "Auxiliary":string, "Heater Auto":string, "Percentage Heat":string, "Temperature Set Point":string, "PID Auto (from file)":string, "P Value":string, "I Value":string, "D Value":string, "Auto PID Table Filename":string, "Flow Auto":string, "Target Heater Table":string, "Sweep mode":string, "Sweep Table Filename":string, "Percentage Flow":string}
  T46 = typedef "Mercury iXX.lvlib/Temperature.lvlib/Temperature Signals Cluster.ctl" = cluster{"Voltage":string, "Current":string, "Power":string, "Resistance":string, "Temperature":string, "Sensitivity":string, "Reference":string}
  T47 = typedef "Mercury iXX.lvlib/Pressure.lvlib/Pressure Device (Read).ctl" = cluster{"Manufacturing":T8, "Temperature Sensor Type":T48, "Calibration":T49, "Control Loop":T51, "Pressure Signals":T11, "Nickname":string, "Status":string}
  T48 = typedef "Mercury iXX.lvlib/Pressure.lvlib/Pressure Sensor Type.ctl" = string
  T49 = typedef "Mercury iXX.lvlib/Pressure.lvlib/Calibration Cluster.ctl" = cluster{"Filename":string, "Interpolation":T50, "Scaling Factor":string, "Offset Factor":string, "High Limit":string, "Low Limit":string, "Last Calibration":string}
  T50 = typedef "Mercury iXX.lvlib/Pressure.lvlib/Calibration Interpolation.ctl" = string
  T51 = typedef "Mercury iXX.lvlib/Pressure.lvlib/Loop Cluster.ctl" = cluster{"Heater":string, "Auxiliary":string, "Heater Auto":string, "Percentage Heat":string, "Pressure Set Point":string, "PID Auto (from file)":string, "P Value":string, "I Value":string, "D Value":string, "Auto PID Table Filename":string, "Flow Auto":string, "Target Heater Table":string, "Sweep mode":string, "Sweep Table Filename":string, "Percentage Flow":string}
  T52 = typedef "Mercury iXX.lvlib/Magnet.lvlib/Output Configuration.ctl" = string
  T53 = typedef "Targets.ctl" = cluster{"Target Field (T)":dbl, "Target Field Rate (T/min)":dbl}
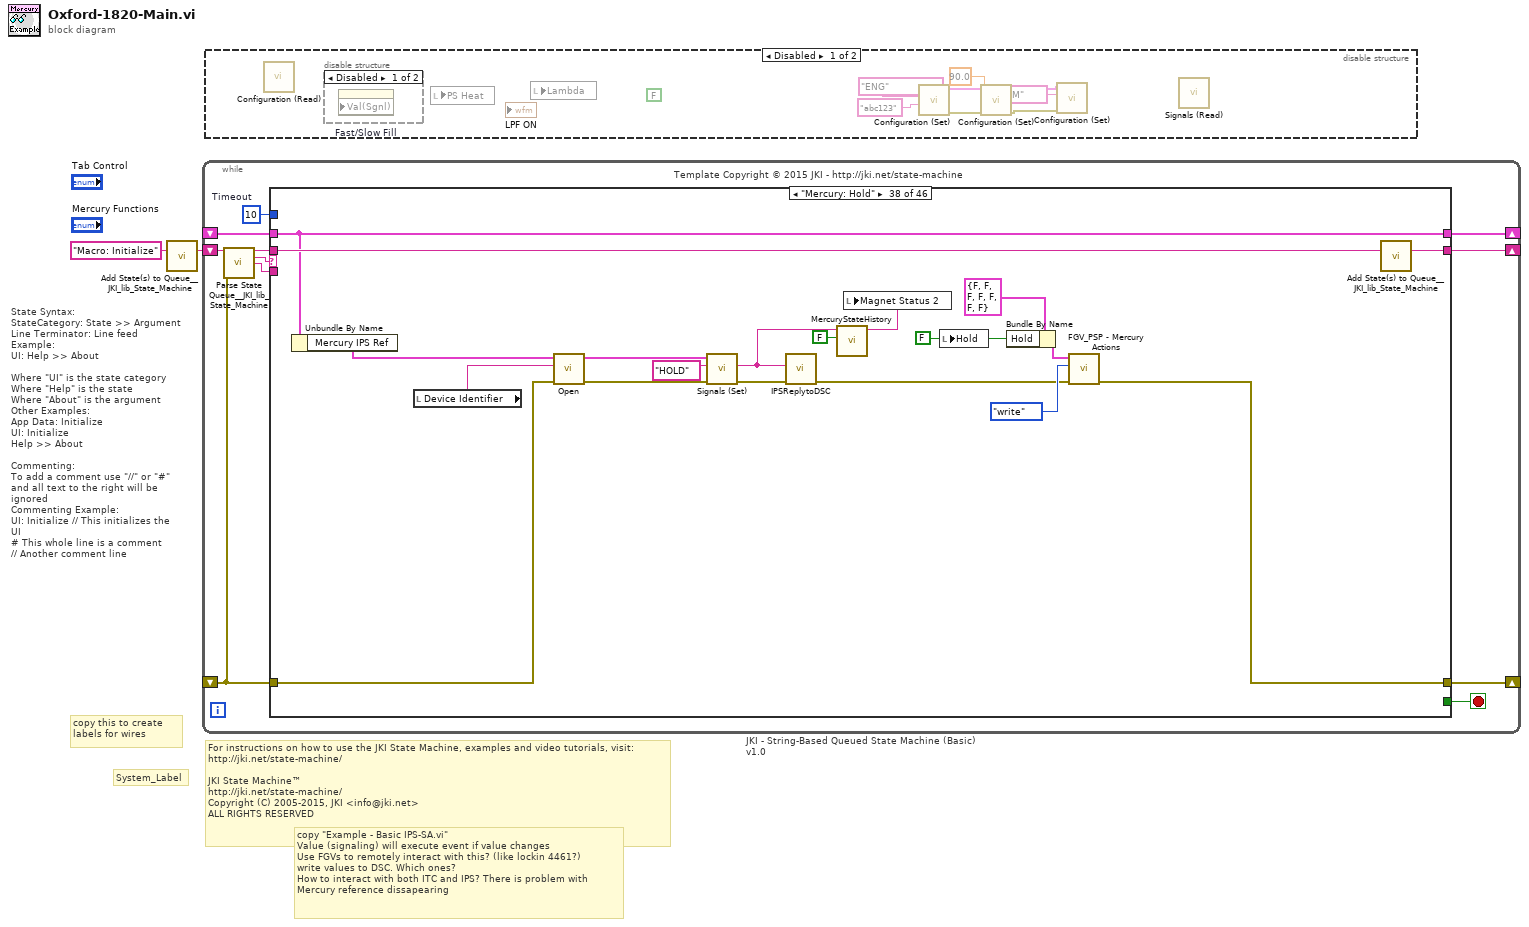
[diagram p0: block diagram]
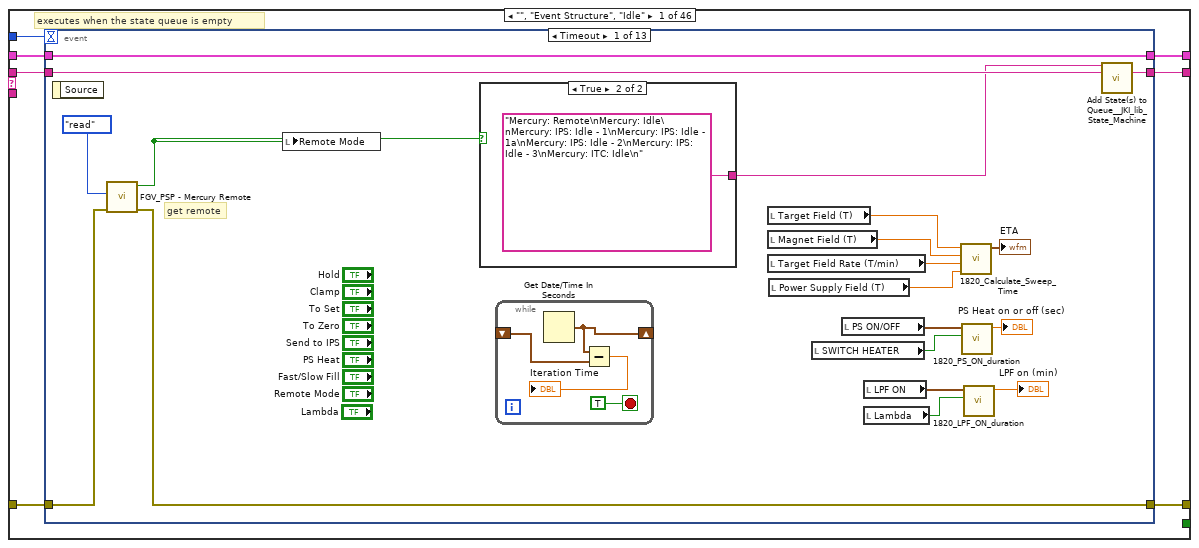
[diagram p4: hidden frame]
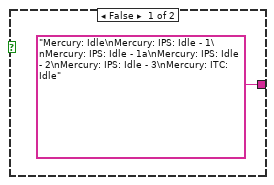
[diagram p5: hidden frame]
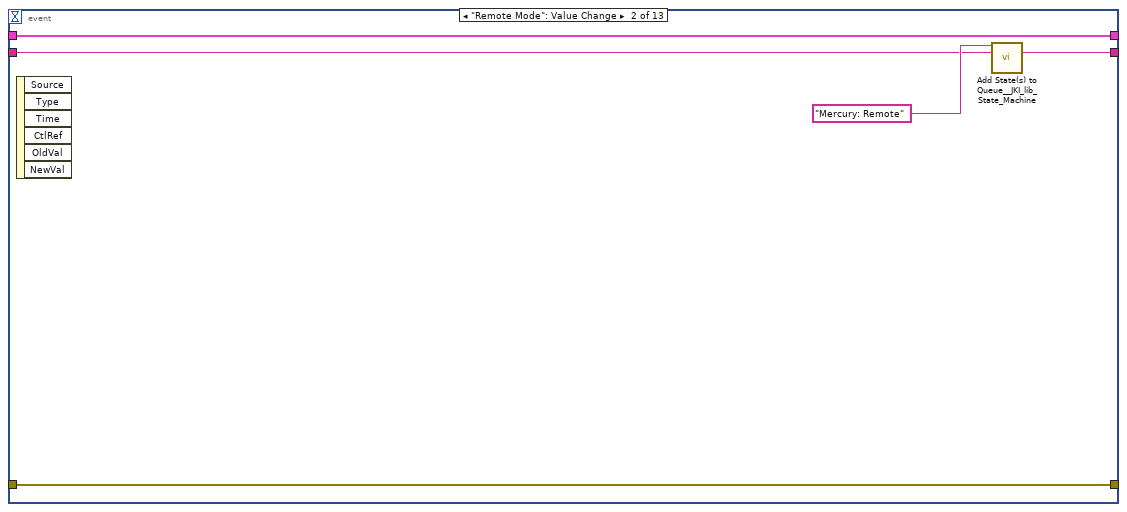
[diagram p6: hidden frame]
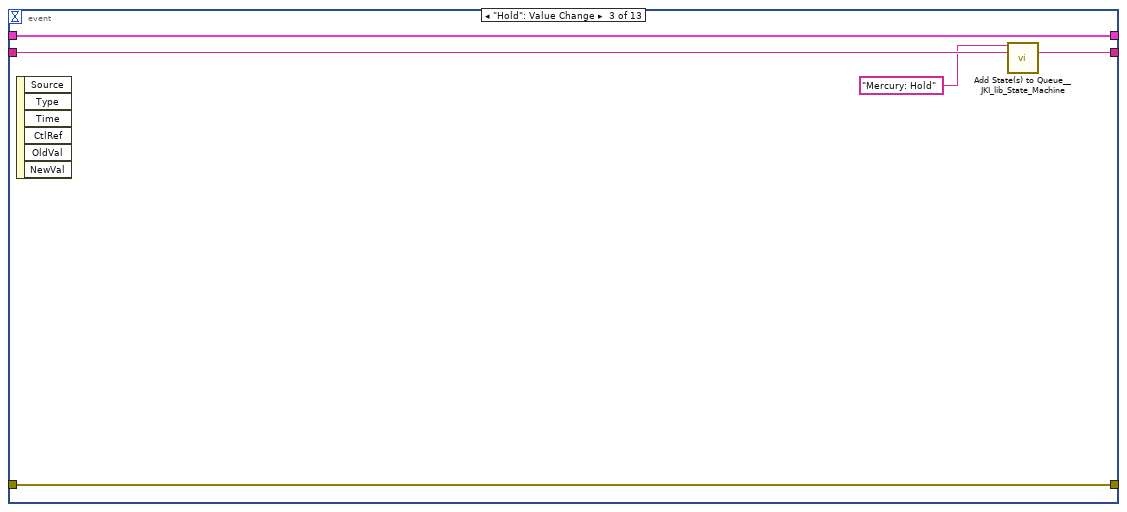
[diagram p7: hidden frame]
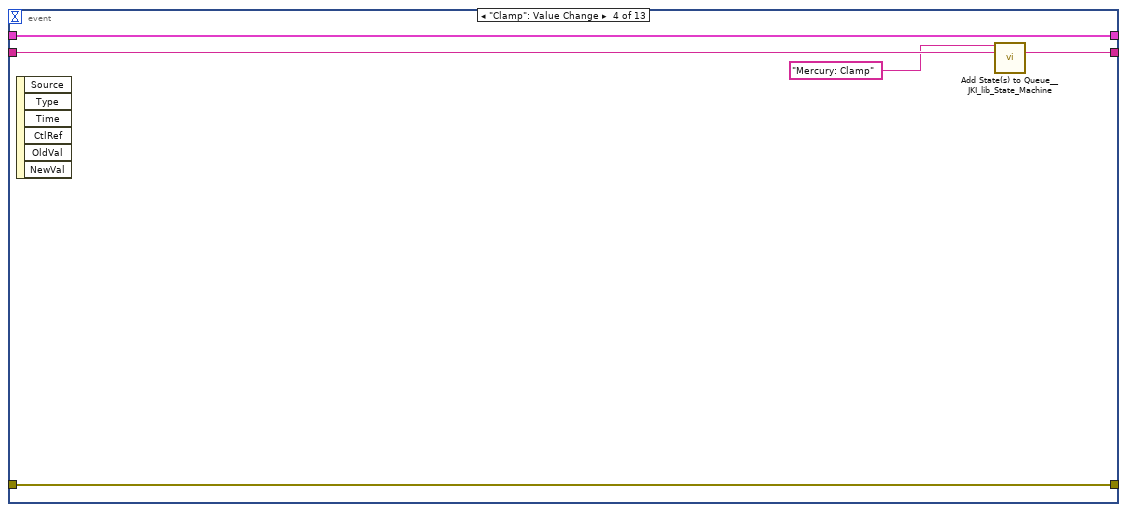
[diagram p8: hidden frame]
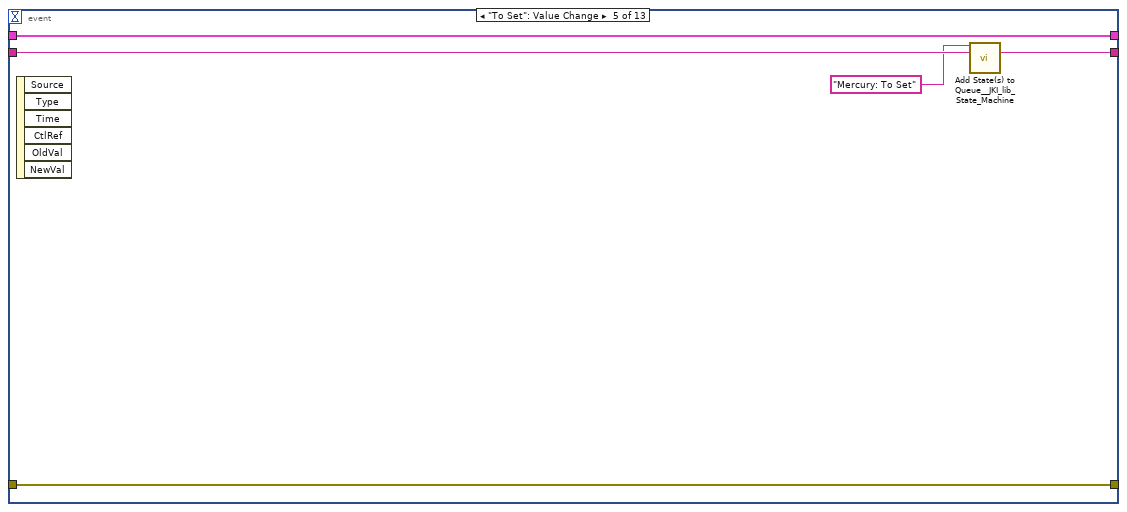
[diagram p9: hidden frame]
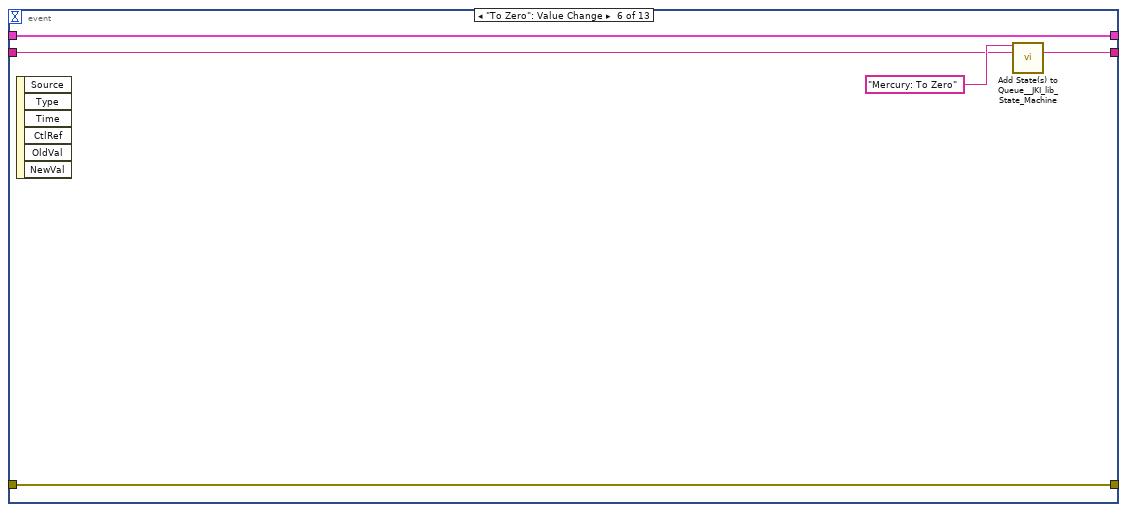
[diagram p10: hidden frame]
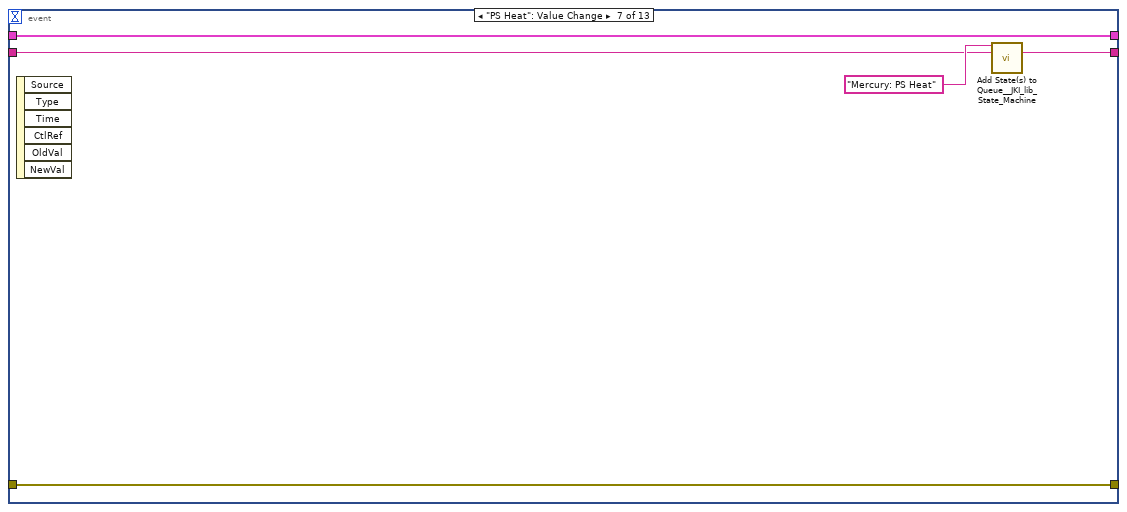
[diagram p11: hidden frame]
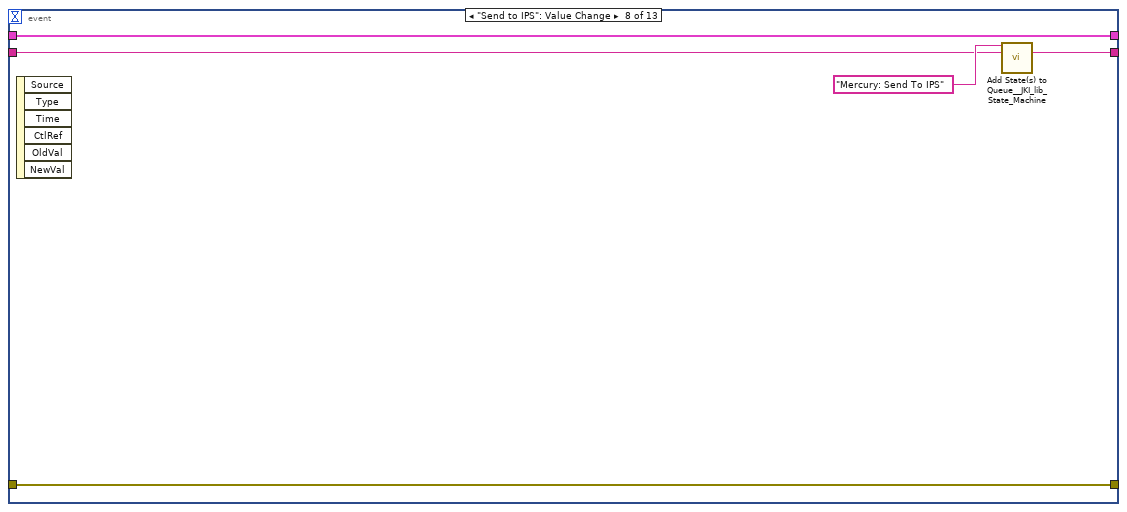
[diagram p12: hidden frame]
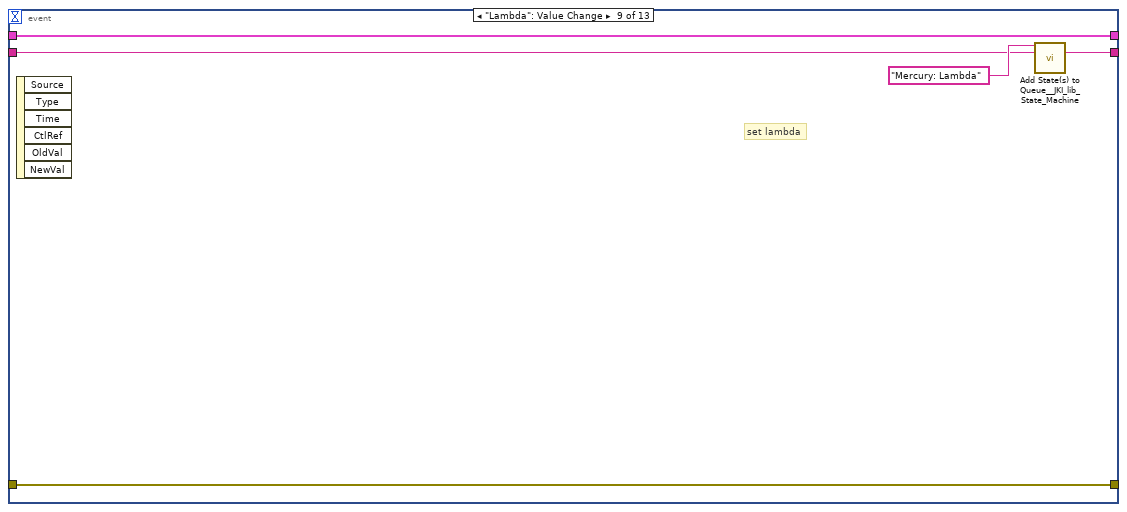
[diagram p13: hidden frame]
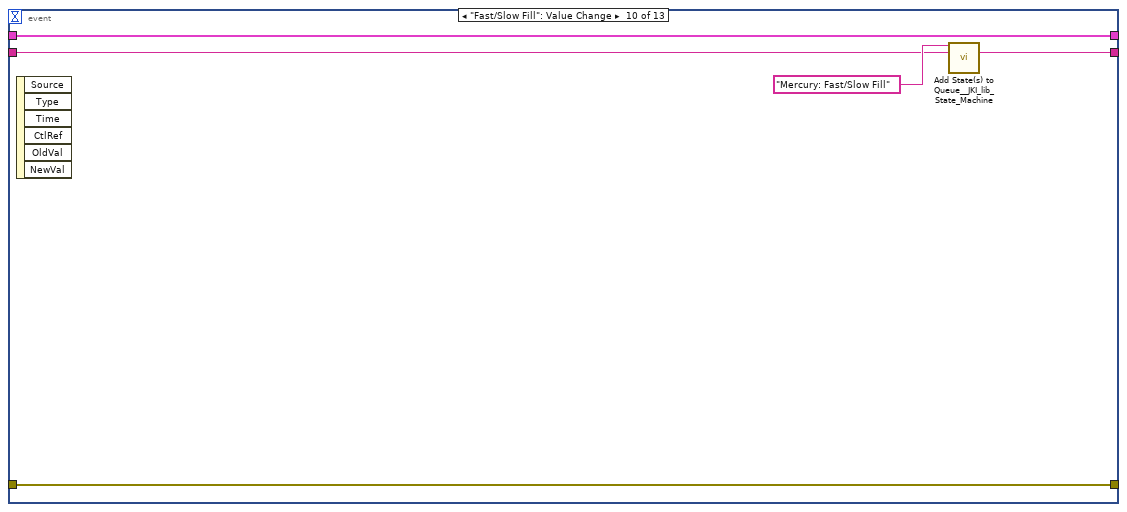
[diagram p14: hidden frame]
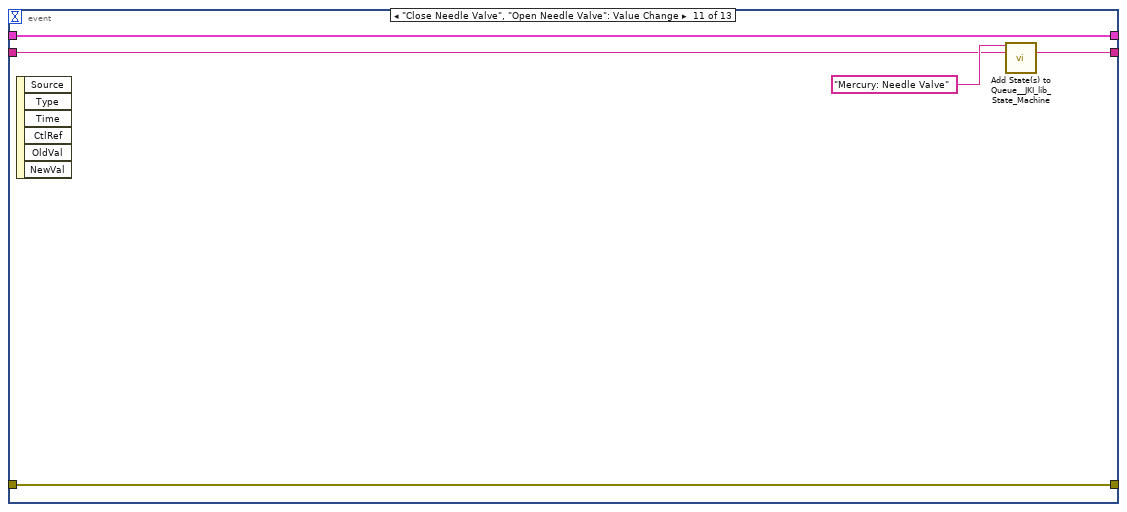
[diagram p15: hidden frame]
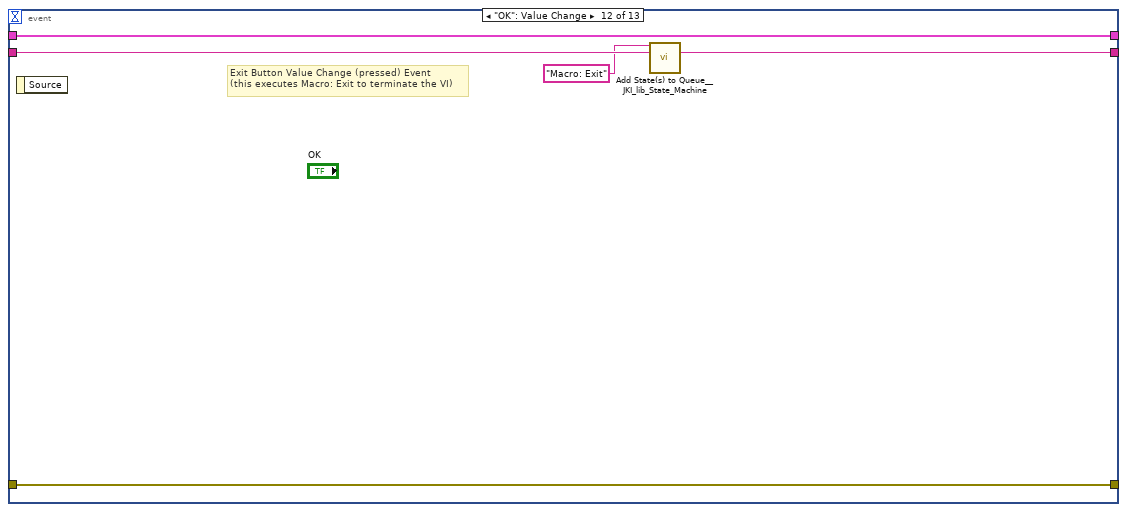
[diagram p16: hidden frame]
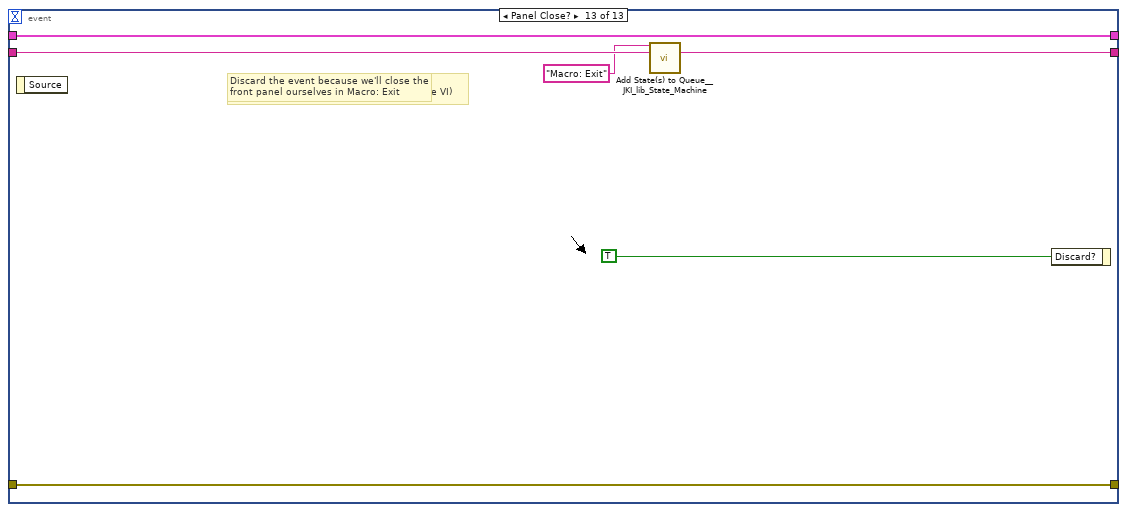
[diagram p17: hidden frame]
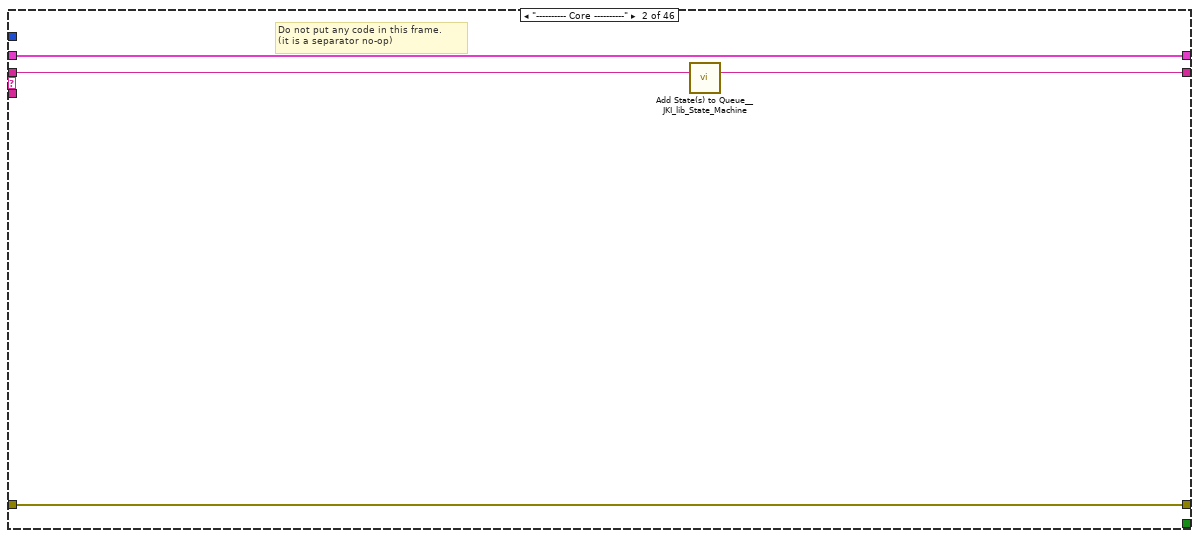
[diagram p18: hidden frame]
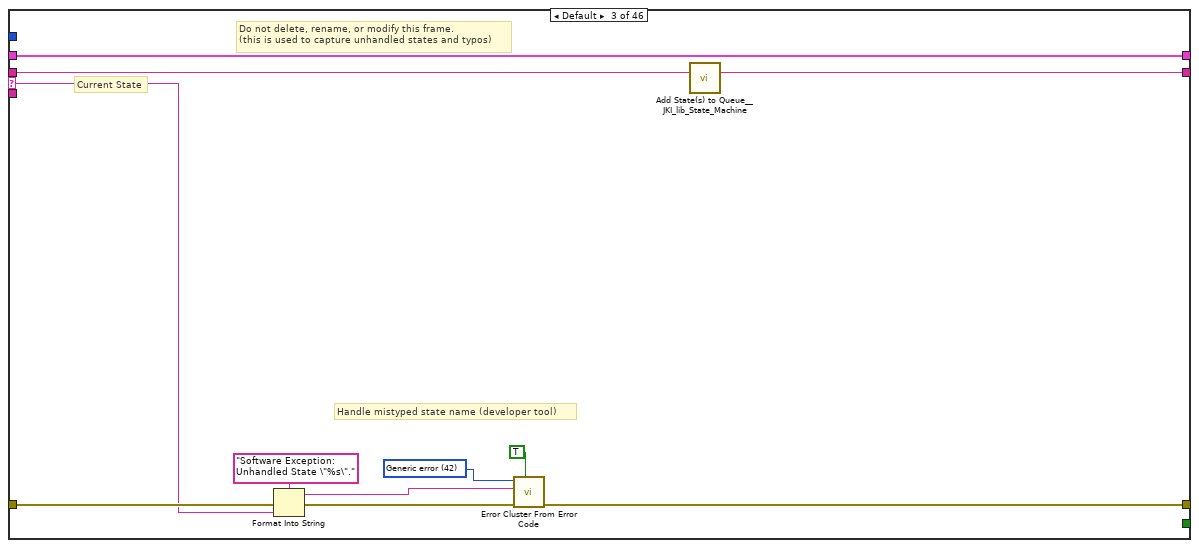
[diagram p19: hidden frame]
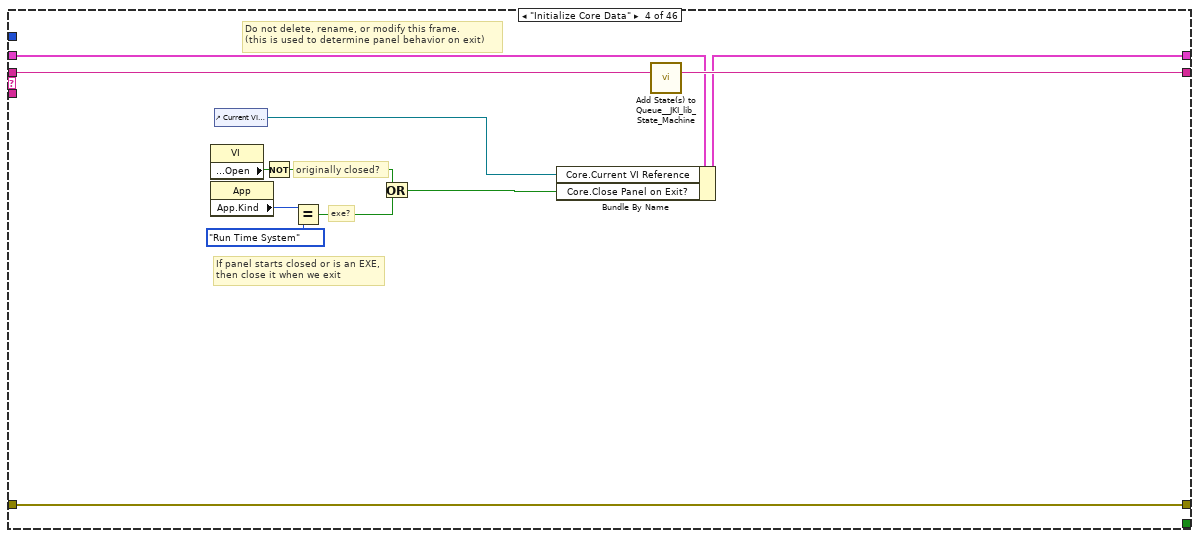
[diagram p20: hidden frame]
diagram:
  # "copy \"Example - Basic IPS-SA.vi\"\nValue (signaling) will execute event if value changes\nUse FGVs to remotely interact with this? (like lockin 4461?)\nwrite values to DSC. Which ones?\nHow to interact with both ITC and IPS? There is problem with \nMercury reference dissapearing"
  # "For instructions on how to use the JKI State Machine, examples and video tutorials, visit:\nhttp://jki.net/state-machine/\n\nJKI State Machine™\nhttp://jki.net/state-machine/\nCopyright (C) 2005-2015, JKI <info@jki.net>\nALL RIGHTS RESERVED"
  # "State Syntax:\nStateCategory: State >> Argument\nLine Terminator: Line feed\nExample:\nUI: Help >> About\n\nWhere \"UI\" is the state category\nWhere \"Help\" is the state\nWhere \"About\" is the argument\nOther Examples:\nApp Data: Initialize\nUI: Initialize\nHelp >> About\n\nCommenting:\nTo add a comment use \"//\" or \"#\" and all text to the right will be ignored\nCommenting Example:\nUI: Initialize // This initializes the UI\n# This whole line is a comment\n// Another comment line"
  # "copy this to create labels for wires"
  # "System_Label"
  n1 = call <vilib>:"Add State(s) to Queue__JKI_lib_State_Machine.vi"("State(s) in (\"\")"="Macro: Initialize") -> ("States Out"=w2:string)  [unwired: 14 in]
  n2 = while "JKI - String-Based Queued State Machine (Basic) v1.0" {
    shift-right: [w6] -> _
    shift-left: _ -> [w5]
    shift-right: [w9] -> _
    shift-left: _ -> [w3]
    shift-right: [w8] -> _
    shift-left: w2 -> [w10]
    stop <- w7 stop-if-true
    w4 = 10  # Timeout
    # "Template Copyright © 2015 JKI - http://jki.net/state-machine"
    n3 = call <vilib>:"Parse State Queue__JKI_lib_State_Machine.vi"("State Queue"=w10, "Error In (no error)"=w3) -> ("Remaining States"=w12:string, "Current State"=w13:string, "Arguments"=w11:string)  [unwired: 11 in]
    n4 = case shown="\"Mercury: Hold\"" w13 {
      selector: w13 -> [_ _ w111 _ _ _ _ _ _ _ _ _ _ _ _ _ _ _ _ _ _ _ _ _ _ _ _ _ _ _ _ _ _ _ _ _ _ _ _ _ _ _ _ _ _ _]
      tunnel: w12 -> [w20 w110 w115 w133 w150 w155 w159 w171 w177 w181 w191 w201 w212 w238 w243 w258 w262 w285 w335 w381 w423 w470 w493 w538 w579 w626 w667 w672 w697 w760 w797 w855 w870 w894 w898 w903 w946 w979 w998 w1017 w1036 w1058 w1126 w1147 w1169 w1186]
      tunnel: w11 -> [_ _ _ _ _ _ _ _ _ _ _ w196 w206 _ _ _ _ _ _ _ _ _ _ _ _ _ _ _ _ _ _ _ _ _ _ _ _ _ _ _ _ _ _ _ _ _]
      tunnel: w5 -> [w16 w107 w113 w124 w136 w153 w156 _ w172 w178 w187 w199 w208 w235 w241 w256 w259 w280 w333 w380 w387 w430 w479 w536 w578 w625 w666 w669 w679 w728 w796 w812 w869 w893 w897 w900 w944 w968 w987 w1006 w1025 w1043 w1111 w1134 w1152 w1173]
      tunnel: [w14 w108 w117 w130 errorcluster {"status"=FALSE, "code"=0, "source"=""} ("error out") w152 w157 w165 w173 w179 w184 w197 w209 w236 w240 w246 w260 w263 w295 w336 w384 w433 w480 w500 w545 w598 w633 w670 w682 w729 w768 w808 w867 w878 w896 w901 w912 w962 w982 w1000 w1019 w1044 w1102 w1128 w1154 w1172] -> w9
      tunnel: [w19 w109 w114 w132 w149 w154 w158 w170 w176 w180 w190 w200 w211 w237 w242 w257 w261 w284 w334 w382 w424 w471 w494 w537 w580 w627 w668 w671 w698 w761 w798 w856 w871 w895 w899 w902 w947 w980 w999 w1018 w1037 w1059 w1127 w1148 w1170 w1187] -> w8
      tunnel: [_ _ _ _ _ TRUE _ _ _ _ _ _ _ _ _ _ _ _ _ _ _ _ _ _ _ _ _ _ _ _ _ _ _ _ _ _ _ _ _ _ _ _ _ _ _ _] -> w7
      tunnel: [w18 w107 w113 w131 w135 w153 w156 w169 w172 w178 w187 w199 w208 w235 w241 w256 w259 w279 w333 w380 w387 w430 w479 w536 w578 w625 w666 w669 w678 w728 w796 w812 w869 w893 w897 w900 w944 w968 w987 w1006 w1025 w1043 w1111 w1134 w1152 w1173] -> w6
      tunnel: w4 -> [w17 _ _ _ _ _ _ _ _ _ _ _ _ _ _ _ _ _ _ _ _ _ _ _ _ _ _ _ _ _ _ _ _ _ _ _ _ _ _ _ _ _ _ _ _ _]
      tunnel: w3 -> [w15 w108 w116 w130 w145 w152 w157 w165 w174 w179 w188 w198 w210 w236 w240 w248 w260 w272 w297 w347 w390 w432 w474 w502 w547 w585 w628 w670 w694 w759 w794 w845 w868 w872 w896 w901 w941 w974 w993 w1012 w1031 w1045 w1121 w1135 w1155 w1171]
      frame "", "Event Structure", "Idle" {
        # "executes when the state queue is empty"
        n5 = event shown="[0] Timeout" {
          selector: _ -> [_ _ _ _ _ _ _ _ _ _ _ _ _]
          dyn-events: _ -> [_ _ _ _ _ _ _ _ _ _ _ _ _]
          timeout: w17 -> [_ _ _ _ _ _ _ _ _ _ _ _ _]
          tunnel: w20 -> [w39 w49 w55 w60 w64 w69 w74 w78 w84 w88 w92 w100 w106]
          tunnel: [w38 w48 w54 w59 w63 w68 w73 w77 w83 w87 w91 w99 w105] -> w19
          tunnel: [w21 w47 w51 w56 w61 w66 w71 w76 w81 w90 w95 w97 w103] -> w18
          tunnel: w16 -> [w21 w47 w51 w56 w61 w66 w71 w76 w81 w90 w95 w97 w103]
          tunnel: w15 -> [w24 w46 w52 w58 w65 w67 w72 w80 w82 w86 w94 w98 w104]
          tunnel: [w23 w46 w52 w58 w65 w67 w72 w80 w82 w86 w94 w98 w104] -> w14
          event Timeout {
            # "get remote"
            n6 = event-data() -> ()  [unwired: 1 in, 1 out]
            n7 = call "FGV_PSP - Mercury Remote.vi"("error in"=w24, "Function"=enum16{"write", "read"}."read") -> ("error out"=w23:errorcluster, "Remote"=w22:bool)  [unwired: 4 in]
            n8 = local write "Remote Mode"(w22) -> ()
            n9 = case shown="True" w22 {
              tunnel: ["Mercury: Idle\nMercury: IPS: Idle - 1\nMercury: IPS: Idle - 1a\nMercury: IPS: Idle - 2\nMercury: IPS: Idle - 3\nMercury: ITC: Idle" ("State(s) at Back (\"\")") "Mercury: Remote\nMercury: Idle\nMercury: IPS: Idle - 1\nMercury: IPS: Idle - 1a\nMercury: IPS: Idle - 2\nMercury: IPS: Idle - 3\nMercury: ITC: Idle\n" ("State(s) at Back (\"\")")] -> w27
              frame False {
              }
              frame True {
              }
            }
            n10 = while {
              shift-right: [w42] -> _
              shift-left: _ -> [w43]
              stop <- TRUE stop-if-true
              n11 = Get Date/Time In Seconds() -> (seconds since 1Jan1904=w42:timestamp)
              n12 = Subtract(x=w42, y=w43) -> (x-y=→"Iteration Time":dbl)
            }
            n13 = local read "Target Field (T)"() -> (w34:dbl)
            n14 = local read "Magnet Field (T)"() -> (w35:dbl)
            n15 = local read "Target Field Rate (T/min)"() -> (w37:dbl)
            n16 = local read "Power Supply Field (T)"() -> (w33:dbl)
            n17 = local read "SWITCH HEATER"() -> (w29:bool)
            n18 = local read "PS ON/OFF"() -> (w30:timestamp)
            n19 = local read "LPF ON"() -> (w32:timestamp)
            n20 = local read "Lambda"() -> (w26:bool)
            n21 = call "1820_Calculate_Sweep_Time.vi"("Power Supply Field (T)"=w33, "Target Field Rate (T/min)"=w37, "Magnet Field (T)"=w35, "Target Field (T)"=w34) -> ("ETA"=→"ETA":timestamp)  [unwired: 6 in, 1 out]
            n22 = call "1820_PS_ON_duration.vi"("SWITCH HEATER"=w29, "time stamp"=w30) -> ("PS Heat on (sec)"=→"PS Heat on or off (sec)":dbl)  [unwired: 9 in]
            n23 = call "1820_LPF_ON_duration.vi"("Lambda"=w26, "LPF ON"=w32) -> ("LPF on (min)"=→"LPF on (min)":dbl)  [unwired: 9 in]
            n24 = call <vilib>:"Add State(s) to Queue__JKI_lib_State_Machine.vi"("State(s) in Front (\"\")"=w27, "State(s) in (\"\")"=w39) -> ("States Out"=w38:string)  [unwired: 13 in]
          }
          event "Remote Mode": Value Change {
            n25 = event-data() -> ()  [unwired: 1 in, 6 out]
            n26 = call <vilib>:"Add State(s) to Queue__JKI_lib_State_Machine.vi"("State(s) in Front (\"\")"="Mercury: Remote", "State(s) in (\"\")"=w49) -> ("States Out"=w48:string)  [unwired: 13 in]
          }
          event "Hold": Value Change {
            n27 = event-data() -> ()  [unwired: 1 in, 6 out]
            n28 = call <vilib>:"Add State(s) to Queue__JKI_lib_State_Machine.vi"("State(s) in Front (\"\")"="Mercury: Hold" ("State(s) in Front (\"\")"), "State(s) in (\"\")"=w55) -> ("States Out"=w54:string)  [unwired: 13 in]
          }
          event "Clamp": Value Change {
            n29 = event-data() -> ()  [unwired: 1 in, 6 out]
            n30 = call <vilib>:"Add State(s) to Queue__JKI_lib_State_Machine.vi"("State(s) in Front (\"\")"="Mercury: Clamp" ("State(s) in Front (\"\")"), "State(s) in (\"\")"=w60) -> ("States Out"=w59:string)  [unwired: 13 in]
          }
          event "To Set": Value Change {
            n31 = event-data() -> ()  [unwired: 1 in, 6 out]
            n32 = call <vilib>:"Add State(s) to Queue__JKI_lib_State_Machine.vi"("State(s) in Front (\"\")"="Mercury: To Set" ("State(s) in Front (\"\")"), "State(s) in (\"\")"=w64) -> ("States Out"=w63:string)  [unwired: 13 in]
          }
          event "To Zero": Value Change {
            n33 = event-data() -> ()  [unwired: 1 in, 6 out]
            n34 = call <vilib>:"Add State(s) to Queue__JKI_lib_State_Machine.vi"("State(s) in Front (\"\")"="Mercury: To Zero" ("State(s) in Front (\"\")"), "State(s) in (\"\")"=w69) -> ("States Out"=w68:string)  [unwired: 13 in]
          }
          event "PS Heat": Value Change {
            n35 = event-data() -> ()  [unwired: 1 in, 6 out]
            n36 = call <vilib>:"Add State(s) to Queue__JKI_lib_State_Machine.vi"("State(s) in Front (\"\")"="Mercury: PS Heat" ("State(s) in Front (\"\")"), "State(s) in (\"\")"=w74) -> ("States Out"=w73:string)  [unwired: 13 in]
          }
          event "Send to IPS": Value Change {
            n37 = event-data() -> ()  [unwired: 1 in, 6 out]
            n38 = call <vilib>:"Add State(s) to Queue__JKI_lib_State_Machine.vi"("State(s) in Front (\"\")"="Mercury: Send To IPS" ("State(s) in Front (\"\")"), "State(s) in (\"\")"=w78) -> ("States Out"=w77:string)  [unwired: 13 in]
          }
          event "Lambda": Value Change {
            # "set lambda"
            n39 = event-data() -> ()  [unwired: 1 in, 6 out]
            n40 = call <vilib>:"Add State(s) to Queue__JKI_lib_State_Machine.vi"("State(s) in Front (\"\")"="Mercury: Lambda" ("State(s) in Front (\"\")"), "State(s) in (\"\")"=w84) -> ("States Out"=w83:string)  [unwired: 13 in]
          }
          event "Fast/Slow Fill": Value Change {
            n41 = event-data() -> ()  [unwired: 1 in, 6 out]
            n42 = call <vilib>:"Add State(s) to Queue__JKI_lib_State_Machine.vi"("State(s) in Front (\"\")"="Mercury: Fast/Slow Fill" ("State(s) in Front (\"\")"), "State(s) in (\"\")"=w88) -> ("States Out"=w87:string)  [unwired: 13 in]
          }
          event "Close Needle Valve", "Open Needle Valve": Value Change {
            n43 = event-data() -> ()  [unwired: 1 in, 6 out]
            n44 = call <vilib>:"Add State(s) to Queue__JKI_lib_State_Machine.vi"("State(s) in Front (\"\")"="Mercury: Needle Valve" ("State(s) in Front (\"\")"), "State(s) in (\"\")"=w92) -> ("States Out"=w91:string)  [unwired: 13 in]
          }
          event "OK": Value Change {
            # "Exit Button Value Change (pressed) Event\n(this executes Macro: Exit to terminate the VI)"
            n45 = event-data() -> ()  [unwired: 1 in, 1 out]
            n46 = call <vilib>:"Add State(s) to Queue__JKI_lib_State_Machine.vi"("State(s) in Front (\"\")"="Macro: Exit", "State(s) in (\"\")"=w100) -> ("States Out"=w99:string)  [unwired: 13 in]
          }
          event Panel Close? {
            # "Discard the event because we'll close the front panel ourselves in Macro: Exit"
            # "Close Panel button (pressed) Event\n(this executes Macro: Exit to terminate the VI)"
            n47 = event-data() -> ()  [unwired: 1 in, 1 out]
            n48 = call <vilib>:"Add State(s) to Queue__JKI_lib_State_Machine.vi"("State(s) in Front (\"\")"="Macro: Exit", "State(s) in (\"\")"=w106) -> ("States Out"=w105:string)  [unwired: 13 in]
            n49 = event-data("Discard?"=TRUE) -> ()  [unwired: 1 in, 1 out]
          }
        }
      }
      frame "---------- Core ----------" {
        # "Do not put any code in this frame.\n(it is a separator no-op)"
        n50 = call <vilib>:"Add State(s) to Queue__JKI_lib_State_Machine.vi"("State(s) in (\"\")"=w110) -> ("States Out"=w109:string)  [unwired: 14 in]
      }
      frame Default {
        w120 = 42 items=["No error", "Argument error", "Memory is full", "Out of zone", "End of file", "File already open", "Generic file I/O error", "File not found", "File permission error", "Disk is full", "Duplicate path", "Too many files open", "System feature not enabled", "Resource file not found", "Cannot add resource", "Resource not found", "Image not found", "Image memory error", "Pen does not exist", "Config type invalid", "Config token not found", "Config parse error", "Config memory error", "Bad external code format", "Bad external code offset", "External code not present", "Null window", "Destroy window error", "Null menu", "Print aborted", "Bad print record", "Print driver error", "Windows error during printing", "Memory error during printing", "Print dialog error", "Generic print error", "Invalid device refnum", "Device not found", "Device parameter error", "Device unit error", "Cannot open device", "Device call aborted", "Generic error", "Cancelled by user", "Object ID too low", "Object ID too high", "Object not in heap", "Unknown heap", "Unknown object (invalid DefProc)", "Unknown object (DefProc not in table)", "Message out of range", "Invalid (null) method", "Unknown message", "Manager call not supported", "Bad address", "Network operation in progress", "Network operation timed out", "Connection is busy", "Network attribute not supported", "Network error", "Address in use", "System out of memory", "Connection aborted", "Connection refused", "Not connected", "Already connected", "Connection closed", "Initialization error (interapplication manager)", "Bad occurrence", "Wait on unbound occurrence handler", "Occurrence queue overflow", "Datalog type conflict", "Unused", "Unrecognized type (interapplication manager)", "Memory corrupt", "Failed to make temporary DLL", "Old CIN version", "Drag socket not found", "Failed to load drop-object", "Failed to register OLE object", "Failed to release OLE object", "Format specifier type mismatch", "Unknown format specifier", "Too few format specifiers", "Too many format specifiers", "Scan failed", "Newer CIN version", "Error converting to variant", "Runtime menu error", "Password tampered", "Variant attribute not found", "Incompatible variant data type", "Event data is not available", "Event Store is not present", "Occurrence is not found", "Event Queue is not created", "Event info is not available", "Refnum passed is NULL", "Error retrieving Class GUID", "Error retrieving CoClass GUID", "Error retrieving TypeLib GUID.", "Bad built application magic bytes.", "Specific driver is different from the specific driver associated with the Logical Name.", "There is no session opened to the class driver.", "Max Error", "MAX - Error with config objects", "MAX - Error loading configuration", "MAX - Group not supported"]
        # "Current State"
        # "Do not delete, rename, or modify this frame.\n(this is used to capture unhandled states and typos)"
        # "Handle mistyped state name (developer tool)"
        n51 = Format Into String(format string="Software Exception: Unhandled State \"%s\"." ("message"), error in=w116, w111) -> (resulting string=w119:string, error out=w118:errorcluster)  [unwired: 1 in]
        n52 = call <vilib>:"Error Cluster From Error Code.vi"("show call chain? (False)"=TRUE, "error in (no error)"=w118, "error message (\"\")"=w119, "error code (0)"=w120) -> ("error out"=w117:errorcluster)  [unwired: 5 in]
        n53 = call <vilib>:"Add State(s) to Queue__JKI_lib_State_Machine.vi"("State(s) in (\"\")"=w115) -> ("States Out"=w114:string)  [unwired: 14 in]
      }
      frame "Initialize Core Data" {
        # "Do not delete, rename, or modify this frame.\n(this is used to determine panel behavior on exit)"
        # "originally closed?"
        # "exe?"
        # "If panel starts closed or is an EXE, then close it when we exit"
        n54 = property class="VI"() -> ("Front Panel.Open"=w129:bool)  [unwired: 2 in, 2 out]
        n55 = property class="App"() -> ("App.Kind"=w128:T26)  [unwired: 2 in, 2 out]
        n56 = control-ref of="Current VI Reference"() -> (w122:refnum<vi>)
        n57 = Not(x=w129) -> (.not. x?=w126:bool)
        n58 = Equal?(x=w128, y=T26."Run Time System" ("Application:Kind")) -> (x = y?=w125:bool)
        n59 = Or(x=w126, y=w125) -> (x .or. y?=w123:bool)
        n60 = Bundle By Name(cluster=w124, "Core.Current VI Reference"=w122, "Core.Close Panel on Exit?"=w123) -> (w131:T39)
        n61 = call <vilib>:"Add State(s) to Queue__JKI_lib_State_Machine.vi"("State(s) in (\"\")"=w133) -> ("States Out"=w132:string)  [unwired: 14 in]
      }
      frame "Error Handler" {
        w144 = i32[] [-1950679035, -1950678943]  # Error Codes to Filter
        # "Unhandled Error -- Display it"
        # "Handle any errors here.\nYou can also output any states to clean-up after errors occur"
        # "Clear error"
        n62 = call-poly <userlib>:"Filter Error Codes__ogtk.vi"("Error In"=w145, "Error Codes to Filter"=w144) -> ("Error Out"=w146:errorcluster, "Filtered Error Details"=w143:T40)  [unwired: 7 in, 1 out]
        n63 = Unbundle(w143) -> ("code"=w141:i32, "source"=w142:string)
        n64 = Get Date/Time In Seconds() -> (seconds since 1Jan1904=w140:timestamp)
        n65 = Unbundle By Name(w136) -> ("Error Log"=w138:T25)
        n66 = Bundle By Name(cluster=T27 {"time"=timestamp(0 s since 1904-01-01), "code"=0, "source"=""} ("output cluster"), "time"=w140, "code"=w141, "source"=w142) -> (w137:T27)
        n67 = Build Array (concatenate)(w138, w137) -> (w134:T25)
        "Error List" <- w134
        n68 = Bundle By Name(cluster=w136, "Error Log"=w134) -> (w135:T39)
        n69 = call <vilib>:"General Error Handler.vi"("error in (no error)"=w146) -> ()  [unwired: 10 in, 5 out]
        n70 = call <vilib>:"Add State(s) to Queue__JKI_lib_State_Machine.vi"("State(s) in Front (\"\")"="/* Post Error States", "State(s) in (\"\")"=w150) -> ("States Out"=w149:string)  [unwired: 13 in]
      }
      frame "Exit" {
        # "Do not put any code in this frame.\n(No errors that occur here will be handled.)"
        n71 = call <vilib>:"Add State(s) to Queue__JKI_lib_State_Machine.vi"("State(s) in (\"\")"=w155) -> ("States Out"=w154:string)  [unwired: 14 in]
      }
      frame "---------- Data ----------" {
        # "Do not put any code in this frame.\n(It is a separator no-op. You can make a copy of this frame to create a new Data frame)"
        n72 = call <vilib>:"Add State(s) to Queue__JKI_lib_State_Machine.vi"("State(s) in (\"\")"=w159) -> ("States Out"=w158:string)  [unwired: 14 in]
      }
      frame "Data: Initialize" {
        w160 = 0  # counter
        w162 = TRUE  # read ITC T?
        w163 = T36 {"Comms"="", "Device ID"=[], "Comms Layer"=enum."Ethernet TCP/IP", "Command"="", "Query reference"=refnum}  # Mercury ITC Ref
        w164 = T25 []  # Error Log
        w166 = TRUE  # sentinel
        w167 = T36 {"Comms"="", "Device ID"=[], "Comms Layer"=enum."Ethernet TCP/IP", "Command"="", "Query reference"=refnum}  # Mercury IPS Ref
        w168 = T41 {"Current VI Reference"=refnum, "Close Panel on Exit?"=FALSE}  # Core
        # "read FGV in timeout"
        # "do not delete - used by framework"
        # "Data names and types of shift register data are defined by this bundle."
        # "Initialize the shift-register data, here.\n(data names are defined by what you wire into the bundle function)"
        n73 = call <vilib>:"Add State(s) to Queue__JKI_lib_State_Machine.vi"("State(s) in (\"\")"=w171) -> ("States Out"=w170:string)  [unwired: 14 in]
        n74 = call "MercuryStateHistory.vi"("initialize?"=TRUE) -> ()  [unwired: 9 in, 2 out]
        n75 = Bundle("Core"=w168, "Mercury ITC Ref"=w163, "Mercury IPS Ref"=w167, "sentinel"=w166, "Error Log"=w164, "read ITC T?"=w162, "counter"=w160) -> (w169:T39)  [unwired: 1 in]
      }
      frame "Data: Cleanup" {
        # "Cleanup any data and references, here.\n(this is called automatically, by the Macro: Exit)"
        n76 = Unbundle By Name(w172) -> ("Core.Current VI Reference"=w175:refnum<vi>)
        n77 = Close Reference(reference=w175, error in (no error)=w174) -> (error out=w173:errorcluster)
        n78 = call <vilib>:"Add State(s) to Queue__JKI_lib_State_Machine.vi"("State(s) in (\"\")"=w177) -> ("States Out"=w176:string)  [unwired: 14 in]
      }
      frame "---------- UI ----------" {
        # "Do not put any code in this frame.\n(It is a separator no-op. You can make a copy of this frame to create a new UI frame)"
        n79 = call <vilib>:"Add State(s) to Queue__JKI_lib_State_Machine.vi"("State(s) in (\"\")"=w181) -> ("States Out"=w180:string)  [unwired: 14 in]
      }
      frame "UI: Initialize" {
        w185 = FALSE
        # "start in local mode"
        # "Initialize the User Interface, here.\n(this is called automatically, by the Macro: Init)"
        n80 = disable-structure shown="Disabled" {
          frame Disabled {
            n81 = Open Application Reference() -> (0:w193:errorcluster, 3:w192:refnum<vi>)  [unwired: 4 in]
            n82 = Open VI Reference(vi path=path "") -> ()  [unwired: 5 in, 2 out]
            n83 = property class="App"(reference=w192, error in=w193, "WebSrvr.Active"=TRUE ("Web Server:Server Active")) -> ()  [unwired: 2 out]
            n84 = call "MNK_Dashboard_v2.vi"() -> ()  [unwired: 12 in]
          }
          frame Enabled {
          }
        }
        n85 = call <userlib>:"Fit VI window to Largest Dec__ogtk.vi"("error in (no error)"=w188) -> ("error out"=w186:errorcluster)  [unwired: 5 in, 1 out]
        n86 = call <vilib>:"Add State(s) to Queue__JKI_lib_State_Machine.vi"("State(s) in (\"\")"=w191) -> ("States Out"=w190:string)  [unwired: 14 in]
        n87 = Number To Boolean Array(number=0.0 ("x")) -> (Boolean array=w183:bool[])
        n88 = local write "LEDs"(w183) -> ()
        n89 = local write "Remote Mode"(w185) -> ()
        n90 = call "FGV_PSP - Mercury Remote.vi"("error in"=w186, "Remote"=w185) -> ("error out"=w184:errorcluster)  [unwired: 4 in, 1 out]
        "Magnet Status 2" <- "" ("Magnet Status 2")
      }
      frame "UI: Cursor Set" {
        # "Argument"
        # "Set and Unset Cursor Busy.\n(Usage: \"UI: Cursor Set >> Busy|Idle\")"
        n91 = case shown="\"Idle\", Default" w196 {
          tunnel: w198 -> [w203 w205]
          tunnel: [w202 w204] -> w197
          frame "Idle", Default {
            n92 = call <vilib>:"Unset Busy.vi"("error in (no error)"=w203) -> ("error out"=w202:errorcluster)  [unwired: 10 in]
          }
          frame "Busy" {
            n93 = call <vilib>:"Set Busy.vi"("error in (no error)"=w205) -> ("error out"=w204:errorcluster)  [unwired: 9 in, 1 out]
          }
        }
        n94 = call <vilib>:"Add State(s) to Queue__JKI_lib_State_Machine.vi"("State(s) in (\"\")"=w201) -> ("States Out"=w200:string)  [unwired: 14 in]
      }
      frame "UI: Front Panel State" {
        # "Argument"
        # "Set Front Panel Open or Closed\n(Usage: \"UI: Front Panel State >> Open|Close\")"
        n95 = Unbundle By Name(w208) -> ("Core.Current VI Reference"=w207:refnum<vi>)
        n96 = case shown="\"Open\", Default" w206 {
          tunnel: w210 -> [w216 w229]
          tunnel: [w218 w230] -> w209
          tunnel: w207 -> [w217 w227]
          frame "Open", Default {
            n97 = property class="VI"(reference=w217, error in=w216) -> (reference out=w214:refnum<vi>, error out=w215:errorcluster, "Front Panel.Open"=w213:bool)
            n98 = case shown="True" w213 {
              tunnel: [w221 w224] -> w218
              tunnel: w215 -> [w220 w224]
              tunnel: w214 -> [w219 _]
              frame False {
                n99 = invoke class="VI" method="FP.Open"(reference=w219, error in=w220, "Activate"=TRUE, "State"=T28."Standard") -> (error out=w221:errorcluster)  [unwired: 1 in, 4 out]
              }
              frame True {
              }
            }
          }
          frame "Close" {
            n100 = property class="VI"(reference=w227, error in=w229) -> (reference out=w226:refnum<vi>, error out=w228:errorcluster, "Front Panel.Open"=w225:bool)
            n101 = case shown="True" w225 {
              tunnel: [w231 w234] -> w230
              tunnel: w228 -> [w231 w233]
              tunnel: w226 -> [_ w232]
              frame False {
              }
              frame True {
                n102 = invoke class="VI" method="FP.Close"(reference=w232, error in=w233) -> (error out=w234:errorcluster)  [unwired: 1 in, 2 out]
              }
            }
          }
        }
        n103 = call <vilib>:"Add State(s) to Queue__JKI_lib_State_Machine.vi"("State(s) in (\"\")"=w212) -> ("States Out"=w211:string)  [unwired: 14 in]
      }
      frame "---------- Macro ----------" {
        # "Do not put any code in this frame.\n(It is a separator no-op. You can make a copy of this frame to create a new Macro frame)"
        n104 = call <vilib>:"Add State(s) to Queue__JKI_lib_State_Machine.vi"("State(s) in (\"\")"=w238) -> ("States Out"=w237:string)  [unwired: 14 in]
      }
      frame "Macro: Initialize" {
        w239 = "Data: Initialize\nInitialize Core Data\nUI: Initialize\nUI: Front Panel State >> Open\nMercury: Initialize"  # Data: Initialize Initialize Core Data UI: Initialize UI: Front Panel State >> Open Mercury: Initialize
        # "Initialization Macro\n(This is called once, when the VI starts)"
        n105 = call <vilib>:"Add State(s) to Queue__JKI_lib_State_Machine.vi"("State(s) in Front (\"\")"=w239, "State(s) in (\"\")"=w243) -> ("States Out"=w242:string)  [unwired: 13 in]
      }
      frame "Macro: Exit" {
        # "Exit Macro\n(This is called once, when the VI exits)"
        n106 = Unbundle By Name(w256) -> ("Core.Close Panel on Exit?"=w255:bool, "Mercury ITC Ref"=w244:T36, "Mercury IPS Ref"=w245:T36)
        n107 = call <instrlib>:"Close.vi"("error in (no error)"=w248, "Mercury Reference"=w245) -> ("error out"=w247:errorcluster)  [unwired: 9 out]
        n108 = call <instrlib>:"Close.vi"("error in (no error)"=w247, "Mercury Reference"=w244) -> ("error out"=w249:errorcluster)  [unwired: 9 out]
        n109 = call <vilib>:"Simple Error Handler.vi"("error in (no error)"=w249) -> ("error out"=w246:errorcluster)  [unwired: 1 in, 7 out]
        n110 = Select(t="UI: Front Panel State >> Close", s=w255, f="") -> (s? t:f=w252:string)
        n111 = call <vilib>:"Add State(s) to Queue__JKI_lib_State_Machine.vi"("State(s) in (\"\")"=w252, "State(s) at Back (\"\")"="Data: Cleanup\nExit") -> ("States Out"=w250:string)  [unwired: 13 in]
        n112 = call <vilib>:"Add State(s) to Queue__JKI_lib_State_Machine.vi"("State(s) in Front (\"\")"=w250, "State(s) in (\"\")"=w258) -> ("States Out"=w257:string)  [unwired: 13 in]
      }
      frame "---------- Mercury: Query ----------" {
        n113 = call <vilib>:"Add State(s) to Queue__JKI_lib_State_Machine.vi"("State(s) in (\"\")"=w262) -> ("States Out"=w261:string)  [unwired: 14 in]
      }
      frame "Mercury: Initialize" {
        w271 = Comms_Transport_Layer."Ethernet TCP/IP" ("Comms Layer")
        n114 = call-poly <instrlib>:"Open.vi"("Clear Previous Connections (False)"=TRUE ("Clear Previous Connections (True)"), "ID Query (True)"=TRUE, "IP Address"="ITC IP Address", "error in (no error)"=w272, "Comms Layer"=w271) -> ("error out"=w266:errorcluster, "# of Instruments"=→"# of Instruments":i32, "Serial Number(s)"=→"Serial Number(s)":string[], "Mercury Reference Out"=w267:T36, "S/W Version(s)"=→"S/W Version(s)":string[])  [unwired: 2 in]
        n115 = call-poly <instrlib>:"Open.vi"("Clear Previous Connections (False)"=FALSE ("Clear Previous Connections (True)"), "ID Query (True)"=TRUE, "IP Address"="IPS IP Address", "error in (no error)"=w266, "Comms Layer"=w271) -> ("error out"=w263:errorcluster, "# of Instruments"=→"# of Instruments 2":i32, "Serial Number(s)"=→"Serial Number(s) 2":string[], "Mercury Reference Out"=w265:T36, "S/W Version(s)"=→"S/W Version(s) 2":string[])  [unwired: 2 in]
        n116 = Bundle By Name(cluster=w280, "Mercury ITC Ref"=w267, "Mercury IPS Ref"=w265) -> (w279:T39)
        n117 = case shown="No Error" w263 {
          tunnel: ["Mercury: Query ITC: System\nMercury: Query IPS: System\nMercury: Query ITC: Temperature\nMercury: Query ITC: Heater\nMercury: Query ITC: Aux\nMercury: Query ITC: Pressure\nMercury: Query IPS: LVL\nMercury: Query IPS: Temperature\nMercury: Query IPS: Magnet" ("State(s) at Back (\"\")") "Error Handler\nMacro: Exit" ("State(s) at Back (\"\")")] -> w264
          frame No Error {
            n118 = Power Of 2(x=9.0) -> (2^x=w287:dbl)
            n119 = Decrement(x=w287) -> (x-1=w288:dbl)
            n120 = Number To Boolean Array(number=w288) -> (Boolean array=w289:bool[])
            n121 = local write "LEDs"(w289) -> ()
          }
          frame Error {
          }
        }
        n122 = call <vilib>:"Add State(s) to Queue__JKI_lib_State_Machine.vi"("State(s) in Front (\"\")"=w264, "State(s) in (\"\")"=w285) -> ("States Out"=w284:string)  [unwired: 13 in]
      }
      frame "Mercury: Query ITC: System" {
        n123 = Unbundle By Name(w333) -> ("Mercury ITC Ref"=w293:T36)
        n124 = call-poly <instrlib>:"Configuration (Read).vi"("error in"=w297, "Mercury Reference In"=w293) -> ("error out"=w329:errorcluster, "Devices"=→"ITC Devices":string[], "Mercury Reference Out"=w330:T36)  [unwired: 1 in, 6 out]
        n125 = call-poly <instrlib>:"Configuration (Read).vi"("error in"=w329, "Mercury Reference In"=w330) -> ("error out"=w322:errorcluster, "Automatic Dimming"=→"Automatic Dimming":string, "Mercury Reference Out"=w323:T36)  [unwired: 1 in, 6 out]
        n126 = call-poly <instrlib>:"Configuration (Read).vi"("error in"=w322, "Mercury Reference In"=w323) -> ("error out"=w325:errorcluster, "Dimming Time"=→"Dimming Time":string, "Mercury Reference Out"=w324:T36)  [unwired: 1 in, 6 out]
        n127 = call-poly <instrlib>:"Configuration (Read).vi"("error in"=w325, "Mercury Reference In"=w324) -> ("error out"=w331:errorcluster, "Display Brightness"=→"Display Brightness":string, "Mercury Reference Out"=w332:T36)  [unwired: 1 in, 6 out]
        n128 = call-poly <instrlib>:"Configuration (Read).vi"("error in"=w331, "Mercury Reference In"=w332) -> ("error out"=w316:errorcluster, "Date"=→"Date":string, "Mercury Reference Out"=w315:T36)  [unwired: 1 in, 6 out]
        n129 = call-poly <instrlib>:"Configuration (Read).vi"("error in"=w316, "Mercury Reference In"=w315) -> ("error out"=w318:errorcluster, "Time"=→"Time":string, "Mercury Reference Out"=w317:T36)  [unwired: 1 in, 6 out]
        n130 = call-poly <instrlib>:"Configuration (Read).vi"("error in"=w318, "Mercury Reference In"=w317) -> ("error out"=w296:errorcluster, "time stamp"=→"time stamp":timestamp, "Mercury Reference Out"=w294:T36)  [unwired: 1 in, 6 out]
        n131 = call-poly <instrlib>:"Configuration (Read).vi"("error in"=w296, "Mercury Reference In"=w294) -> ("error out"=w314:errorcluster, "Hardware Version"=→"Hardware Version":string, "Mercury Reference Out"=w313:T36)  [unwired: 1 in, 6 out]
        n132 = call-poly <instrlib>:"Configuration (Read).vi"("error in"=w314, "Mercury Reference In"=w313) -> ("error out"=w312:errorcluster, "Firmware Version"=→"Firmware Version":string, "Mercury Reference Out"=w311:T36)  [unwired: 1 in, 6 out]
        n133 = call-poly <instrlib>:"Configuration (Read).vi"("error in"=w312, "Mercury Reference In"=w311) -> ("error out"=w299:errorcluster, "Serial Number"=→"Serial Number":string, "Mercury Reference Out"=w298:T36)  [unwired: 1 in, 6 out]
        n134 = call-poly <instrlib>:"Configuration (Read).vi"("error in"=w299, "Mercury Reference In"=w298) -> ("error out"=w305:errorcluster, "Free Space"=→"Free Space":i32, "Mercury Reference Out"=w304:T36)  [unwired: 1 in, 6 out]
        n135 = call-poly <instrlib>:"Configuration (Read).vi"("error in"=w305, "Mercury Reference In"=w304) -> ("error out"=w301:errorcluster, "Mode"=→"String":T42, "Mercury Reference Out"=w302:T36)  [unwired: 1 in, 6 out]
        n136 = Get Date/Time In Seconds() -> (seconds since 1Jan1904=w310:timestamp)
        n137 = call-poly <instrlib>:"Configuration (Set).vi"("error in"=w301, "time stamp"=w310, "Mercury Reference In"=w302) -> ("error out"=w295:errorcluster, "Response"=→"Set Date Response":T35)  [unwired: 1 in, 6 out]
        n138 = call <vilib>:"Add State(s) to Queue__JKI_lib_State_Machine.vi"("State(s) in (\"\")"=w335) -> ("States Out"=w334:string)  [unwired: 14 in]
      }
      frame "Mercury: Query ITC: Temperature" {
        # "Temperature"
        n139 = Unbundle By Name(w380) -> ("Mercury ITC Ref"=w342:T36)
        n140 = local read "ITC Devices"() -> (w341:string[])
        n141 = Index Array(array=w341, index=3) -> (element=w343:string)
        n142 = call-poly <instrlib>:"Open.vi"("error in (no error)"=w347, "Device Identifier"=w343, "Mercury Reference In"=w342) -> ("error out"=w359:errorcluster, "Mercury Reference Out"=w360:T36)  [unwired: 7 out]
        n143 = call-poly <instrlib>:"Configuration (Read).vi"("error in"=w359, "Mercury Reference In"=w360) -> ("error out"=w351:errorcluster, "Serial Number"=→"Temp S/N":string, "Mercury Reference Out"=w350:T36)  [unwired: 1 in, 6 out]
        n144 = call-poly <instrlib>:"Configuration (Read).vi"("error in"=w351, "Mercury Reference In"=w350) -> ("error out"=w353:errorcluster, "Nickname"=→"T Nickname":string, "Mercury Reference Out"=w352:T36)  [unwired: 1 in, 6 out]
        n145 = call-poly <instrlib>:"Configuration (Read).vi"("error in"=w353, "Mercury Reference In"=w352) -> ("error out"=w356:errorcluster, "Unit"=→"Unit":T3, "Excitation Magnitude"=→"Excitation Magnitude":dbl, "Mercury Reference Out"=w355:T36)  [unwired: 1 in, 5 out]
        n146 = call-poly <instrlib>:"Configuration (Read).vi"("error in"=w356, "Mercury Reference In"=w355) -> ("error out"=w346:errorcluster, "Sensor Type"=→"Sensor Type":T43, "Mercury Reference Out"=w344:T36)  [unwired: 1 in, 6 out]
        n147 = call-poly <instrlib>:"Configuration (Read).vi"("error in"=w346, "Mercury Reference In"=w344) -> ("error out"=w362:errorcluster, "Excitation Type"=→"Excitation Type":T7, "Mercury Reference Out"=w363:T36)  [unwired: 1 in, 6 out]
        n148 = call-poly <instrlib>:"Configuration (Read).vi"("error in"=w362, "Mercury Reference In"=w363) -> ("error out"=w364:errorcluster, "Unit"=→"H Unit":T3, "Hot Limit"=→"Hot Limit":dbl, "Mercury Reference Out"=w365:T36)  [unwired: 1 in, 5 out]
        n149 = call-poly <instrlib>:"Configuration (Read).vi"("error in"=w364, "Mercury Reference In"=w365) -> ("error out"=w371:errorcluster, "Unit"=→"C Unit":T3, "Cold Limit"=→"Cold Limit":dbl, "Mercury Reference Out"=w370:T36)  [unwired: 1 in, 5 out]
        n150 = call-poly <instrlib>:"Signals (Read).vi"("error in"=w371, "Mercury Reference In"=w370) -> ("error out"=w375:errorcluster, "Unit"=→"V Unit":T3, "Voltage"=→"Voltage":dbl, "Mercury Reference Out"=w374:T36)  [unwired: 1 in, 5 out]
        n151 = call-poly <instrlib>:"Signals (Read).vi"("error in"=w375, "Mercury Reference In"=w374) -> ("error out"=w376:errorcluster, "Unit"=→"T Unit":T3, "Temperature"=→"Temperature":dbl, "Mercury Reference Out"=w379:T36)  [unwired: 1 in, 5 out]
        n152 = call-poly <instrlib>:"Configuration (Read).vi"("error in"=w376, "Mercury Reference In"=w379) -> ("error out"=w336:errorcluster, "Device Details"=w337:T44)  [unwired: 1 in, 7 out]
        n153 = Unbundle By Name(w337) -> ("Manufacturing"=→"ITC Manufacturing":T8, "Excitation"=→"ITC Excitation":T6, "Calibration"=→"ITC Calibration":T4)
        n154 = call <vilib>:"Add State(s) to Queue__JKI_lib_State_Machine.vi"("State(s) in (\"\")"=w381) -> ("States Out"=w382:string)  [unwired: 14 in]
      }
      frame "Mercury: Query ITC: Heater" {
        # "Heater"
        n155 = Unbundle By Name(w387) -> ("Mercury ITC Ref"=w386:T36)
        n156 = local read "ITC Devices"() -> (w388:string[])
        n157 = Index Array(array=w388, index=2) -> (element=w383:string)
        n158 = call-poly <instrlib>:"Open.vi"("error in (no error)"=w390, "Device Identifier"=w383, "Mercury Reference In"=w386) -> ("error out"=w393:errorcluster, "Mercury Reference Out"=w392:T36)  [unwired: 7 out]
        n159 = call-poly <instrlib>:"Configuration (Read).vi"("error in"=w393, "Mercury Reference In"=w392) -> ("error out"=w400:errorcluster, "Device Details"=→"Heater Device Settings":T9, "Mercury Reference Out"=w399:T36)  [unwired: 1 in, 6 out]
        n160 = call-poly <instrlib>:"Configuration (Read).vi"("error in"=w400, "Mercury Reference In"=w399) -> ("error out"=w402:errorcluster, "Nickname"=→"Htr Nickname":string, "Mercury Reference Out"=w401:T36)  [unwired: 1 in, 6 out]
        n161 = call-poly <instrlib>:"Configuration (Read).vi"("error in"=w402, "Mercury Reference In"=w401) -> ("error out"=w395:errorcluster, "Serial Number"=→"Htr S/N":string, "Mercury Reference Out"=w394:T36)  [unwired: 1 in, 6 out]
        n162 = call-poly <instrlib>:"Configuration (Read).vi"("error in"=w395, "Mercury Reference In"=w394) -> ("error out"=w391:errorcluster, "Unit"=→"Volt Unit":T3, "Voltage Limit"=→"Htr Voltage Limit":dbl, "Mercury Reference Out"=w385:T36)  [unwired: 1 in, 5 out]
        n163 = call-poly <instrlib>:"Configuration (Read).vi"("error in"=w391, "Mercury Reference In"=w385) -> ("error out"=w405:errorcluster, "Unit"=→"Res Unit":T3, "Nominal Resistance"=→"Htr Resistance":dbl, "Mercury Reference Out"=w406:T36)  [unwired: 1 in, 5 out]
        n164 = call-poly <instrlib>:"Configuration (Read).vi"("error in"=w405, "Mercury Reference In"=w406) -> ("error out"=w412:errorcluster, "Unit"=→"Power Unit":T3, "Maximum Power"=→"Maximum Power":dbl, "Mercury Reference Out"=w411:T36)  [unwired: 1 in, 5 out]
        n165 = call-poly <instrlib>:"Signals (Read).vi"("error in"=w412, "Mercury Reference In"=w411) -> ("error out"=w414:errorcluster, "Unit"=→"Htr V Unit":T3, "Voltage"=→"Htr Voltage":dbl, "Mercury Reference Out"=w413:T36)  [unwired: 1 in, 5 out]
        n166 = call-poly <instrlib>:"Signals (Read).vi"("error in"=w414, "Mercury Reference In"=w413) -> ("error out"=w416:errorcluster, "Unit"=→"Htr P Unit":T3, "Power"=→"Htr Power":dbl, "Mercury Reference Out"=w415:T36)  [unwired: 1 in, 5 out]
        n167 = call-poly <instrlib>:"Signals (Read).vi"("error in"=w416, "Mercury Reference In"=w415) -> ("error out"=w384:errorcluster, "Unit"=→"Htr C Unit":T3, "Current"=→"Htr Current":dbl)  [unwired: 1 in, 6 out]
        n168 = call <vilib>:"Add State(s) to Queue__JKI_lib_State_Machine.vi"("State(s) in (\"\")"=w423) -> ("States Out"=w424:string)  [unwired: 14 in]
      }
      frame "Mercury: Query ITC: Aux" {
        # "Auxiliary"
        n169 = Unbundle By Name(w430) -> ("Mercury ITC Ref"=w425:T36)
        n170 = local read "ITC Devices"() -> (w428:string[])
        n171 = Index Array(array=w428, index=0) -> (element=w426:string)
        n172 = call-poly <instrlib>:"Open.vi"("error in (no error)"=w432, "Device Identifier"=w426, "Mercury Reference In"=w425) -> ("error out"=w452:errorcluster, "Mercury Reference Out"=w453:T36)  [unwired: 7 out]
        n173 = call-poly <instrlib>:"Configuration (Read).vi"("error in"=w452, "Mercury Reference In"=w453) -> ("error out"=w456:errorcluster, "Auxiliary Device Details"=→"Auxiliary Device Details":T12, "Mercury Reference Out"=w455:T36)  [unwired: 1 in, 6 out]
        n174 = call-poly <instrlib>:"Configuration (Read).vi"("error in"=w456, "Mercury Reference In"=w455) -> ("error out"=w459:errorcluster, "Serial Number"=→"Aux S/N":string, "Mercury Reference Out"=w458:T36)  [unwired: 1 in, 6 out]
        n175 = call-poly <instrlib>:"Configuration (Read).vi"("error in"=w459, "Mercury Reference In"=w458) -> ("error out"=w461:errorcluster, "Unit"=→"Unit 2":T3, "Min Flow"=→"Min Flow":dbl, "Mercury Reference Out"=w460:T36)  [unwired: 1 in, 5 out]
        n176 = call-poly <instrlib>:"Configuration (Read).vi"("error in"=w461, "Mercury Reference In"=w460) -> ("error out"=w463:errorcluster, "Unit"=→"Unit 3":T3, "Scaling Factor"=→"Scaling Factor":dbl, "Mercury Reference Out"=w462:T36)  [unwired: 1 in, 5 out]
        n177 = call-poly <instrlib>:"Configuration (Read).vi"("error in"=w463, "Mercury Reference In"=w462) -> ("error out"=w431:errorcluster, "Unit"=→"Unit 4":T3, "Temp Err"=→"Temp Err":dbl, "Mercury Reference Out"=w427:T36)  [unwired: 1 in, 5 out]
        n178 = call-poly <instrlib>:"Configuration (Read).vi"("error in"=w431, "Mercury Reference In"=w427) -> ("error out"=w435:errorcluster, "Unit"=→"Unit 5":T3, "Temp V Err"=→"Temp V Err":dbl, "Mercury Reference Out"=w434:T36)  [unwired: 1 in, 5 out]
        n179 = call-poly <instrlib>:"Configuration (Read).vi"("error in"=w435, "Mercury Reference In"=w434) -> ("error out"=w437:errorcluster, "Unit"=→"Unit 6":T3, "Gear"=→"Gear":u32, "Mercury Reference Out"=w436:T36)  [unwired: 1 in, 5 out]
        n180 = call-poly <instrlib>:"Configuration (Read).vi"("error in"=w437, "Mercury Reference In"=w436) -> ("error out"=w445:errorcluster, "Unit"=→"Unit 7":T3, "Speed"=→"Speed":u32, "Mercury Reference Out"=w444:T36)  [unwired: 1 in, 5 out]
        n181 = call-poly <instrlib>:"Signals (Read).vi"("error in"=w445, "Mercury Reference In"=w444) -> ("error out"=w447:errorcluster, "Unit"=→"Unit":T3, "Position"=→"Position":u32, "Mercury Reference Out"=w446:T36)  [unwired: 1 in, 5 out]
        n182 = call-poly <instrlib>:"Signals (Read).vi"("error in"=w447, "Mercury Reference In"=w446) -> ("error out"=w433:errorcluster, "Unit"=→"Unit":T3, "% Open"=→"% Open":dbl)  [unwired: 1 in, 6 out]
        n183 = call <vilib>:"Add State(s) to Queue__JKI_lib_State_Machine.vi"("State(s) in (\"\")"=w470) -> ("States Out"=w471:string)  [unwired: 14 in]
      }
      frame "Mercury: Query ITC: Pressure" {
        # "Pressure"
        n184 = Unbundle By Name(w479) -> ("Mercury ITC Ref"=w476:T36)
        n185 = local read "ITC Devices"() -> (w478:string[])
        n186 = Index Array(array=w478, index=1) -> (element=w475:string)
        n187 = call-poly <instrlib>:"Open.vi"("error in (no error)"=w474, "Device Identifier"=w475, "Mercury Reference In"=w476) -> ("error out"=w482:errorcluster, "Mercury Reference Out"=w483:T36)  [unwired: 7 out]
        n188 = call-poly <instrlib>:"Configuration (Read).vi"("error in"=w482, "Mercury Reference In"=w483) -> ("error out"=w484:errorcluster, "Device Details"=w481:T47, "Mercury Reference Out"=w485:T36)  [unwired: 1 in, 6 out]
        n189 = Unbundle By Name(w481) -> ("Manufacturing"=→"Manufacturing":T8, "Pressure Signals"=→"Pressure Signals":T11)
        n190 = call-poly <instrlib>:"Configuration (Read).vi"("error in"=w484, "Mercury Reference In"=w485) -> ("error out"=w489:errorcluster, "Nickname"=→"Nickname":string, "Mercury Reference Out"=w490:T36)  [unwired: 1 in, 6 out]
        n191 = call-poly <instrlib>:"Signals (Read).vi"("error in"=w489, "Mercury Reference In"=w490) -> ("error out"=w487:errorcluster, "Current"=→"Current":dbl, "Mercury Reference Out"=w488:T36)  [unwired: 1 in, 6 out]
        n192 = call-poly <instrlib>:"Signals (Read).vi"("error in"=w487, "Mercury Reference In"=w488) -> ("error out"=w480:errorcluster, "Voltage"=→"Voltage":dbl)  [unwired: 1 in, 7 out]
        n193 = call <vilib>:"Add State(s) to Queue__JKI_lib_State_Machine.vi"("State(s) in (\"\")"=w493) -> ("States Out"=w494:string)  [unwired: 14 in]
      }
      frame "Mercury: Query IPS: System" {
        # "Your code here.\n(You can make a copy of, or modify, this frame)"
        n194 = Unbundle By Name(w536) -> ("Mercury IPS Ref"=w497:T36)
        n195 = call-poly <instrlib>:"Configuration (Read).vi"("error in"=w502, "Mercury Reference In"=w497) -> ("error out"=w522:errorcluster, "Devices"=→"IPS Devices":string[], "Mercury Reference Out"=w521:T36)  [unwired: 1 in, 6 out]
        n196 = call-poly <instrlib>:"Configuration (Read).vi"("error in"=w522, "Mercury Reference In"=w521) -> ("error out"=w526:errorcluster, "Automatic Dimming"=→"Automatic Dimming 2":string, "Mercury Reference Out"=w525:T36)  [unwired: 1 in, 6 out]
        n197 = call-poly <instrlib>:"Configuration (Read).vi"("error in"=w526, "Mercury Reference In"=w525) -> ("error out"=w523:errorcluster, "Dimming Time"=→"Dimming Time 2":string, "Mercury Reference Out"=w524:T36)  [unwired: 1 in, 6 out]
        n198 = call-poly <instrlib>:"Configuration (Read).vi"("error in"=w523, "Mercury Reference In"=w524) -> ("error out"=w520:errorcluster, "Display Brightness"=→"Display Brightness 2":string, "Mercury Reference Out"=w519:T36)  [unwired: 1 in, 6 out]
        n199 = call-poly <instrlib>:"Configuration (Read).vi"("error in"=w520, "Mercury Reference In"=w519) -> ("error out"=w529:errorcluster, "Date"=→"Date 2":string, "Mercury Reference Out"=w530:T36)  [unwired: 1 in, 6 out]
        n200 = call-poly <instrlib>:"Configuration (Read).vi"("error in"=w529, "Mercury Reference In"=w530) -> ("error out"=w527:errorcluster, "Time"=→"Time 2":string, "Mercury Reference Out"=w528:T36)  [unwired: 1 in, 6 out]
        n201 = call-poly <instrlib>:"Configuration (Read).vi"("error in"=w527, "Mercury Reference In"=w528) -> ("error out"=w501:errorcluster, "time stamp"=→"time stamp 2":timestamp, "Mercury Reference Out"=w498:T36)  [unwired: 1 in, 6 out]
        n202 = call-poly <instrlib>:"Configuration (Read).vi"("error in"=w501, "Mercury Reference In"=w498) -> ("error out"=w503:errorcluster, "Hardware Version"=→"Hardware Version 2":string, "Mercury Reference Out"=w504:T36)  [unwired: 1 in, 6 out]
        n203 = call-poly <instrlib>:"Configuration (Read).vi"("error in"=w503, "Mercury Reference In"=w504) -> ("error out"=w505:errorcluster, "Firmware Version"=→"Firmware Version 2":string, "Mercury Reference Out"=w506:T36)  [unwired: 1 in, 6 out]
        n204 = call-poly <instrlib>:"Configuration (Read).vi"("error in"=w505, "Mercury Reference In"=w506) -> ("error out"=w511:errorcluster, "Serial Number"=→"Serial Number 2":string, "Mercury Reference Out"=w512:T36)  [unwired: 1 in, 6 out]
        n205 = call-poly <instrlib>:"Configuration (Read).vi"("error in"=w511, "Mercury Reference In"=w512) -> ("error out"=w507:errorcluster, "Free Space"=→"Free Space 2":i32, "Mercury Reference Out"=w508:T36)  [unwired: 1 in, 6 out]
        n206 = call-poly <instrlib>:"Configuration (Read).vi"("error in"=w507, "Mercury Reference In"=w508) -> ("error out"=w510:errorcluster, "Mode"=→"String 2":T42, "Mercury Reference Out"=w509:T36)  [unwired: 1 in, 6 out]
        n207 = Get Date/Time In Seconds() -> (seconds since 1Jan1904=w518:timestamp)
        n208 = call-poly <instrlib>:"Configuration (Set).vi"("error in"=w510, "time stamp"=w518, "Mercury Reference In"=w509) -> ("error out"=w500:errorcluster, "Response"=→"Set Date Response 2":T35)  [unwired: 1 in, 6 out]
        n209 = call <vilib>:"Add State(s) to Queue__JKI_lib_State_Machine.vi"("State(s) in (\"\")"=w538) -> ("States Out"=w537:string)  [unwired: 14 in]
      }
      frame "Mercury: Query IPS: LVL" {
        # "Level"
        n210 = Unbundle By Name(w578) -> ("Mercury IPS Ref"=w541:T36)
        n211 = local read "IPS Devices"() -> (w577:string[])
        n212 = Index Array(array=w577, index=0) -> (element=w540:string)
        n213 = call-poly <instrlib>:"Open.vi"("error in (no error)"=w547, "Device Identifier"=w540, "Mercury Reference In"=w541) -> ("error out"=w563:errorcluster, "Mercury Reference Out"=w562:T36)  [unwired: 7 out]
        n214 = call-poly <instrlib>:"Configuration (Read).vi"("error in"=w563, "Mercury Reference In"=w562) -> ("error out"=w568:errorcluster, "LVL Device Settings"=→"LVL Device DetailSettings":T14, "Mercury Reference Out"=w565:T36)  [unwired: 1 in, 6 out]
        n215 = call-poly <instrlib>:"Configuration (Read).vi"("error in"=w568, "Mercury Reference In"=w565) -> ("error out"=w569:errorcluster, "Serial Number"=→"LVL S/N":string, "Mercury Reference Out"=w567:T36)  [unwired: 1 in, 6 out]
        n216 = call-poly <instrlib>:"Configuration (Read).vi"("error in"=w569, "Mercury Reference In"=w567) -> ("error out"=w572:errorcluster, "Resistance Configuration"=→"He Res Config":T19, "Mercury Reference Out"=w571:T36)  [unwired: 1 in, 6 out]
        n217 = call-poly <instrlib>:"Configuration (Read).vi"("error in"=w572, "Mercury Reference In"=w571) -> ("error out"=w574:errorcluster, "Magnitude"=→"LVL P Magnitude":dbl, "Mercury Reference Out"=w573:T36)  [unwired: 1 in, 6 out]
        n218 = call-poly <instrlib>:"Configuration (Read).vi"("error in"=w574, "Mercury Reference In"=w573) -> ("error out"=w546:errorcluster, "Duration"=→"LVL P Duration":dbl, "Mercury Reference Out"=w544:T36)  [unwired: 1 in, 6 out]
        n219 = call-poly <instrlib>:"Configuration (Read).vi"("error in"=w546, "Mercury Reference In"=w544) -> ("error out"=w550:errorcluster, "Freq 100%"=→"N Freq 100%":dbl, "Mercury Reference Out"=w549:T36)  [unwired: 1 in, 6 out]
        n220 = call-poly <instrlib>:"Configuration (Read).vi"("error in"=w550, "Mercury Reference In"=w549) -> ("error out"=w553:errorcluster, "Pulse Period"=→"N Pulse Period":dbl, "Mercury Reference Out"=w552:T36)  [unwired: 1 in, 6 out]
        n221 = call-poly <instrlib>:"Signals (Read).vi"("error in"=w553, "Mercury Reference In"=w552) -> ("error out"=w555:errorcluster, "Resistance"=→"He Resistance":dbl, "Mercury Reference Out"=w554:T36)  [unwired: 1 in, 6 out]
        n222 = call-poly <instrlib>:"Signals (Read).vi"("error in"=w555, "Mercury Reference In"=w554) -> ("error out"=w557:errorcluster, "Level"=→"He Level" →"He LEVEL":dbl, "Mercury Reference Out"=w556:T36)  [unwired: 1 in, 6 out]
        n223 = call-poly <instrlib>:"Signals (Read).vi"("error in"=w557, "Mercury Reference In"=w556) -> ("error out"=w559:errorcluster, "Counter"=→"N Counter":u32, "Mercury Reference Out"=w558:T36)  [unwired: 1 in, 6 out]
        n224 = call-poly <instrlib>:"Signals (Read).vi"("error in"=w559, "Mercury Reference In"=w558) -> ("error out"=w545:errorcluster, "Level"=→"N Level" →"N2 LEVEL":dbl)  [unwired: 1 in, 7 out]
        n225 = call <vilib>:"Add State(s) to Queue__JKI_lib_State_Machine.vi"("State(s) in (\"\")"=w579) -> ("States Out"=w580:string)  [unwired: 14 in]
      }
      frame "Mercury: Query IPS: Temperature" {
        n226 = Unbundle By Name(w625) -> ("Mercury IPS Ref"=w586:T36)
        n227 = local read "IPS Devices"() -> (w624:string[])
        n228 = Index Array(array=w624, index=4) -> (element=w587:string)
        n229 = call-poly <instrlib>:"Open.vi"("error in (no error)"=w585, "Device Identifier"=w587, "Mercury Reference In"=w586) -> ("error out"=w612:errorcluster, "Mercury Reference Out"=w607:T36)  [unwired: 7 out]
        n230 = call-poly <instrlib>:"Configuration (Read).vi"("error in"=w612, "Mercury Reference In"=w607) -> ("error out"=w613:errorcluster, "Serial Number"=→"Temp S/N 2":string, "Mercury Reference Out"=w608:T36)  [unwired: 1 in, 6 out]
        n231 = call-poly <instrlib>:"Configuration (Read).vi"("error in"=w613, "Mercury Reference In"=w608) -> ("error out"=w614:errorcluster, "Nickname"=→"T Nickname 2":string, "Mercury Reference Out"=w609:T36)  [unwired: 1 in, 6 out]
        n232 = call-poly <instrlib>:"Configuration (Read).vi"("error in"=w614, "Mercury Reference In"=w609) -> ("error out"=w615:errorcluster, "Unit"=→"Unit 12":T3, "Excitation Magnitude"=→"Excitation Magnitude 2":dbl, "Mercury Reference Out"=w610:T36)  [unwired: 1 in, 5 out]
        n233 = call-poly <instrlib>:"Configuration (Read).vi"("error in"=w615, "Mercury Reference In"=w610) -> ("error out"=w616:errorcluster, "Sensor Type"=→"Sensor Type 2":T43, "Mercury Reference Out"=w611:T36)  [unwired: 1 in, 6 out]
        n234 = call-poly <instrlib>:"Configuration (Read).vi"("error in"=w616, "Mercury Reference In"=w611) -> ("error out"=w589:errorcluster, "Excitation Type"=→"Excitation Type 2":T7, "Mercury Reference Out"=w588:T36)  [unwired: 1 in, 6 out]
        n235 = call-poly <instrlib>:"Configuration (Read).vi"("error in"=w589, "Mercury Reference In"=w588) -> ("error out"=w594:errorcluster, "Unit"=→"H Unit 2":T3, "Hot Limit"=→"Hot Limit 2":dbl, "Mercury Reference Out"=w590:T36)  [unwired: 1 in, 5 out]
        n236 = call-poly <instrlib>:"Configuration (Read).vi"("error in"=w594, "Mercury Reference In"=w590) -> ("error out"=w595:errorcluster, "Unit"=→"C Unit 2":T3, "Cold Limit"=→"Cold Limit 2":dbl, "Mercury Reference Out"=w591:T36)  [unwired: 1 in, 5 out]
        n237 = call-poly <instrlib>:"Signals (Read).vi"("error in"=w595, "Mercury Reference In"=w591) -> ("error out"=w596:errorcluster, "Unit"=→"V Unit 2":T3, "Voltage"=→"Voltage 2":dbl, "Mercury Reference Out"=w592:T36)  [unwired: 1 in, 5 out]
        n238 = call-poly <instrlib>:"Signals (Read).vi"("error in"=w596, "Mercury Reference In"=w592) -> ("error out"=w597:errorcluster, "Unit"=→"T Unit 2":T3, "Temperature"=→"Temperature 2":dbl, "Mercury Reference Out"=w593:T36)  [unwired: 1 in, 5 out]
        n239 = call-poly <instrlib>:"Configuration (Read).vi"("error in"=w597, "Mercury Reference In"=w593) -> ("error out"=w598:errorcluster, "Device Details"=w581:T44)  [unwired: 1 in, 7 out]
        n240 = Unbundle By Name(w581) -> ("Manufacturing"=→"IPS Manufacturing":T8, "Excitation"=→"IPS Excitation":T6, "Calibration"=→"IPS Calibration":T4)
        n241 = call <vilib>:"Add State(s) to Queue__JKI_lib_State_Machine.vi"("State(s) in (\"\")"=w626) -> ("States Out"=w627:string)  [unwired: 14 in]
      }
      frame "Mercury: Query IPS: Magnet" {
        n242 = Unbundle By Name(w666) -> ("Mercury IPS Ref"=w632:T36)
        n243 = call-poly <instrlib>:"Open.vi"("error in (no error)"=w628, "Device Identifier"="Device Identifier", "Mercury Reference In"=w632) -> ("error out"=w651:errorcluster, "Mercury Reference Out"=w650:T36)  [unwired: 7 out]
        n244 = call-poly <instrlib>:"Configuration (Read).vi"("error in"=w651, "Mercury Reference In"=w650) -> ("error out"=w654:errorcluster, "Magnet Device Details"=→"Magnet Device Details":T22, "Mercury Reference Out"=w653:T36)  [unwired: 1 in, 6 out]
        n245 = call-poly <instrlib>:"Configuration (Read).vi"("error in"=w654, "Mercury Reference In"=w653) -> ("error out"=w657:errorcluster, "Serial Number"=→"Mag S/N":string, "Mercury Reference Out"=w656:T36)  [unwired: 1 in, 6 out]
        n246 = call-poly <instrlib>:"Configuration (Read).vi"("error in"=w657, "Mercury Reference In"=w656) -> ("error out"=w660:errorcluster, "Bipolar Output"=→"Bipolar Output":string, "Mercury Reference Out"=w659:T36)  [unwired: 1 in, 6 out]
        n247 = call-poly <instrlib>:"Configuration (Read).vi"("error in"=w660, "Mercury Reference In"=w659) -> ("error out"=w663:errorcluster, "Out Config"=→"Out Config":T52, "Mercury Reference Out"=w662:T36)  [unwired: 1 in, 6 out]
        n248 = call-poly <instrlib>:"Configuration (Read).vi"("error in"=w663, "Mercury Reference In"=w662) -> ("error out"=w634:errorcluster, "Unit"=→"Unit 8":T3, "Current Limit"=→"Current Limit":dbl, "Mercury Reference Out"=w631:T36)  [unwired: 1 in, 5 out]
        n249 = call-poly <instrlib>:"Configuration (Read).vi"("error in"=w634, "Mercury Reference In"=w631) -> ("error out"=w637:errorcluster, "Unit"=→"Unit 9":T3, "AtoB"=→"AtoB":dbl, "Mercury Reference Out"=w636:T36)  [unwired: 1 in, 5 out]
        n250 = call-poly <instrlib>:"Configuration (Read).vi"("error in"=w637, "Mercury Reference In"=w636) -> ("error out"=w640:errorcluster, "Switch Present"=→"Switch Present":string, "Mercury Reference Out"=w639:T36)  [unwired: 1 in, 6 out]
        n251 = call-poly <instrlib>:"Configuration (Read).vi"("error in"=w640, "Mercury Reference In"=w639) -> ("error out"=w645:errorcluster, "Unit"=→"Unit 10":T3, "SW VLIM"=→"SW VLIM":dbl, "Mercury Reference Out"=w644:T36)  [unwired: 1 in, 5 out]
        n252 = call-poly <instrlib>:"Signals (Read).vi"("error in"=w645, "Mercury Reference In"=w644) -> ("error out"=w647:errorcluster, "Unit"=→"Unit 11":T3, "Current Rate"=→"Current Rate":dbl, "Mercury Reference Out"=w646:T36)  [unwired: 1 in, 5 out]
        n253 = call-poly <instrlib>:"Signals (Read).vi"("error in"=w647, "Mercury Reference In"=w646) -> ("error out"=w633:errorcluster, "PSU Act Stat"=→"PSU Act Stat":T32)  [unwired: 1 in, 7 out]
        n254 = call <vilib>:"Add State(s) to Queue__JKI_lib_State_Machine.vi"("State(s) in (\"\")"=w667) -> ("States Out"=w668:string)  [unwired: 14 in]
      }
      frame "---------- Mercury: Idle ----------" {
        n255 = call <vilib>:"Add State(s) to Queue__JKI_lib_State_Machine.vi"("State(s) in (\"\")"=w672) -> ("States Out"=w671:string)  [unwired: 14 in]
      }
      frame "Mercury: Idle" {
        n256 = Unbundle By Name(w679) -> ("counter"=w674:i32, "sentinel"=w677:bool, "Mercury IPS Ref"=w696:T36, "Mercury ITC Ref"=w695:T36)
        n257 = Not(x=w677) -> (.not. x?=w676:bool)
        n258 = Bundle By Name(cluster=w679, "sentinel"=w676) -> (w678:T39)
        n259 = Increment(x=w674) -> (x+1=w675:i32)
        n260 = call "StarTrekIndicator.vi"("Counter"=w675) -> ("Back and Forth"=→"LEDs":bool[])  [unwired: 8 in, 1 out]
        n261 = disable-structure shown="Enabled" {
          disable-tunnel: w695 -> [w715 _]
          disable-tunnel: w694 -> [w714 w717]
          disable-tunnel: [w701 w717] -> w690
          frame Disabled {
            n262 = local read "ITC Devices"() -> (w712:string[])
            n263 = Index Array(array=w712, index=3) -> (element=w705:string)
            n264 = call-poly <instrlib>:"Open.vi"("error in (no error)"=w714, "Device Identifier"=w705, "Mercury Reference In"=w715) -> ("error out"=w711:errorcluster, "Mercury Reference Out"=w709:T36)  [unwired: 7 out]
            n265 = call-poly <instrlib>:"Signals (Read).vi"("error in"=w711, "Mercury Reference In"=w709) -> ("error out"=w708:errorcluster, "Temperature"=→"LPF Temperature":dbl, "Mercury Reference Out"=w707:T36)  [unwired: 1 in, 6 out]
            n266 = call-poly <instrlib>:"Signals (Read).vi"("error in"=w708, "Mercury Reference In"=w707) -> ("error out"=w704:errorcluster, "Resistance"=→"LPF Resistance":dbl, "Mercury Reference Out"=w703:T36)  [unwired: 1 in, 6 out]
            n267 = call-poly <instrlib>:"Configuration (Set).vi"("error in"=w704, "Excitation Magnitude"=0.0, "Mercury Reference In"=w703) -> ("error out"=w701:errorcluster, "Response"=w700:T35)  [unwired: 5 in, 2 out]
            n268 = call "MercuryStateHistory.vi"("Current State in"=w700) -> ("delimited string"=w699:string)  [unwired: 9 in, 1 out]
            n269 = local write "Magnet Status 2"(w699) -> ()
          }
          frame Enabled {
            w716 = -1.0 ("LPF Temperature")
            n270 = local write "LPF Temperature"(w716) -> ()
            n271 = local write "LPF Resistance"(w716) -> ()
          }
        }
        n272 = local read "IPS Devices"() -> (w693:string[])
        n273 = Index Array(array=w693, index=5) -> (element=w691:string)
        n274 = call-poly <instrlib>:"Open.vi"("error in (no error)"=w690, "Device Identifier"=w691, "Mercury Reference In"=w696) -> ("error out"=w687:errorcluster, "Mercury Reference Out"=w688:T36)  [unwired: 7 out]
        n275 = call-poly <instrlib>:"Signals (Read).vi"("error in"=w687, "Mercury Reference In"=w688) -> ("error out"=w680:errorcluster, "Temperature"=→"Magnet Temperature":dbl, "Mercury Reference Out"=w689:T36)  [unwired: 1 in, 6 out]
        n276 = call-poly <instrlib>:"Signals (Read).vi"("error in"=w680, "Mercury Reference In"=w689) -> ("error out"=w683:errorcluster, "Resistance"=→"Magnet Resistance":dbl, "Mercury Reference Out"=w684:T36)  [unwired: 1 in, 6 out]
        n277 = First Call?() -> (First Call?: T/F=w681:bool)
        n278 = case shown="False" w681 {
          tunnel: [w718 w724] -> w682
          tunnel: w684 -> [_ w720]
          tunnel: w683 -> [w718 w719]
          frame False {
          }
          frame True {
            n279 = call-poly <instrlib>:"Configuration (Set).vi"("error in"=w719, "Excitation Magnitude"=20.0, "Mercury Reference In"=w720) -> ("error out"=w724:errorcluster, "Response"=w722:T35)  [unwired: 5 in, 2 out]
            n280 = call "MercuryStateHistory.vi"("Current State in"=w722) -> ("delimited string"=w721:string)  [unwired: 9 in, 1 out]
            n281 = local write "Magnet Status 2"(w721) -> ()
          }
        }
        n282 = call <vilib>:"Add State(s) to Queue__JKI_lib_State_Machine.vi"("State(s) in (\"\")"=w697) -> ("States Out"=w698:string)  [unwired: 14 in]
      }
      frame "Mercury: IPS: Idle - 1" {
        # "set switch status"
        n283 = Unbundle By Name(w728) -> ("Mercury IPS Ref"=w731:T36)
        n284 = local read "Device Identifier"() -> (w744:T24)
        n285 = call-poly <instrlib>:"Configuration (Read).vi"("error in"=w759, "Mercury Reference In"=w731) -> ("error out"=w751:errorcluster, "Time"=w754:string, "Mercury Reference Out"=w752:T36)  [unwired: 1 in, 6 out]
        n286 = local write "Time 2"(w754) -> ()
        n287 = call-poly <instrlib>:"Open.vi"("error in (no error)"=w751, "Device Identifier"=w744, "Mercury Reference In"=w752) -> ("error out"=w750:errorcluster, "Mercury Reference Out"=w749:T36)  [unwired: 7 out]
        n288 = call-poly <instrlib>:"Signals (Read).vi"("error in"=w750, "Mercury Reference In"=w749) -> ("error out"=w726:errorcluster, "Switch Heater Status"=w730:string, "Mercury Reference Out"=w725:T36)  [unwired: 1 in, 6 out]
        n289 = Equal?(x=w730, y="ON") -> (x = y?=→"SWITCH HEATER":bool)
        n290 = call-poly <instrlib>:"Signals (Read).vi"("error in"=w726, "Mercury Reference In"=w725) -> ("error out"=w758:errorcluster, "Current"=→"Current (A)" →"Current (A)":dbl, "Mercury Reference Out"=w756:T36)  [unwired: 1 in, 6 out]
        n291 = call-poly <instrlib>:"Signals (Read).vi"("error in"=w758, "Mercury Reference In"=w756) -> ("error out"=w743:errorcluster, "Voltage"=→"Voltage (V)" →"Voltage (V)":dbl, "Mercury Reference Out"=w742:T36)  [unwired: 1 in, 6 out]
        n292 = call-poly <instrlib>:"Signals (Read).vi"("error in"=w743, "Mercury Reference In"=w742) -> ("error out"=w745:errorcluster, "Field"=→"Power Supply Field (T)":dbl, "Mercury Reference Out"=w748:T36)  [unwired: 1 in, 6 out]
        n293 = call-poly <instrlib>:"Signals (Read).vi"("error in"=w745, "Mercury Reference In"=w748) -> ("error out"=w746:errorcluster, "Target Field Rate"=→"Target Field Rate (T/min)":dbl, "Mercury Reference Out"=w747:T36)  [unwired: 1 in, 6 out]
        n294 = call-poly <instrlib>:"Signals (Read).vi"("error in"=w746, "Mercury Reference In"=w747) -> ("error out"=w741:errorcluster, "Target Field"=→"Target Field (T)":dbl, "Mercury Reference Out"=w740:T36)  [unwired: 1 in, 6 out]
        n295 = call-poly <instrlib>:"Signals (Read).vi"("error in"=w741, "Mercury Reference In"=w740) -> ("error out"=w757:errorcluster, "Persistant Field"=→"Magnet Field (T)" →"Magnet Field (T)":dbl, "Mercury Reference Out"=w755:T36)  [unwired: 1 in, 6 out]
        n296 = call-poly <instrlib>:"Signals (Read).vi"("error in"=w757, "Mercury Reference In"=w755) -> ("error out"=w729:errorcluster, "PSU Act Stat"=w732:T32)  [unwired: 1 in, 7 out]
        n297 = local write "PSU Act Stat"(w732) -> ()
        n298 = case shown="\"HOLD\"" w732 {
          selector: w732 -> [w762 _ _ _ _]
          tunnel: [w762 "Holding" "Ramping to Setpoint" "Ramping to Zero" "Clamped"] -> w739
          frame Default {
          }
          frame "HOLD" {
          }
          frame "RTOS" {
          }
          frame "RTOZ" {
          }
          frame "CLMP" {
          }
        }
        "Magnet Status" <- w739
        n299 = call <vilib>:"Add State(s) to Queue__JKI_lib_State_Machine.vi"("State(s) in (\"\")"=w760) -> ("States Out"=w761:string)  [unwired: 14 in]
      }
      frame "Mercury: IPS: Idle - 1a" {
        n300 = local read "IPS Devices"() -> (w792:string[])
        n301 = Unbundle By Name(w796) -> ("Mercury IPS Ref"=w795:T36)
        n302 = for {
          tunnel: w792 -> [w800] mode=indexing
          tunnel: [w799] -> w791 mode=indexing
          n303 = Match Pattern(string=w800, regular expression=":PSU") -> (before substring=w799:string)  [unwired: 1 in, 3 out]
        }
        n304 = Index Array(array=w791, index #1=6 ("index")) -> (element #1=w793:string, element #2=w789:string, element #3=w790:string)  [unwired: 2 in]
        n305 = call-poly <instrlib>:"Open.vi"("error in (no error)"=w794, "Device Identifier"=w793, "Mercury Reference In"=w795) -> ("error out"=w771:errorcluster, "Mercury Reference Out"=w775:T36)  [unwired: 7 out]
        n306 = call-poly <instrlib>:"Signals (Read).vi"("error in"=w771, "Mercury Reference In"=w775) -> ("error out"=w777:errorcluster, "Current"=→"M1 Current":dbl, "Mercury Reference Out"=w776:T36)  [unwired: 1 in, 6 out]
        n307 = call-poly <instrlib>:"Signals (Read).vi"("error in"=w777, "Mercury Reference In"=w776) -> ("error out"=w769:errorcluster, "Voltage"=→"M1 Voltage":dbl)  [unwired: 1 in, 7 out]
        n308 = call-poly <instrlib>:"Open.vi"("error in (no error)"=w769, "Device Identifier"=w789, "Mercury Reference In"=w795) -> ("error out"=w772:errorcluster, "Mercury Reference Out"=w774:T36)  [unwired: 7 out]
        n309 = call-poly <instrlib>:"Signals (Read).vi"("error in"=w772, "Mercury Reference In"=w774) -> ("error out"=w780:errorcluster, "Current"=→"M2 Current":dbl, "Mercury Reference Out"=w778:T36)  [unwired: 1 in, 6 out]
        n310 = call-poly <instrlib>:"Signals (Read).vi"("error in"=w780, "Mercury Reference In"=w778) -> ("error out"=w767:errorcluster, "Voltage"=→"M2 Voltage":dbl)  [unwired: 1 in, 7 out]
        n311 = call-poly <instrlib>:"Open.vi"("error in (no error)"=w767, "Device Identifier"=w790, "Mercury Reference In"=w795) -> ("error out"=w770:errorcluster, "Mercury Reference Out"=w773:T36)  [unwired: 7 out]
        n312 = call-poly <instrlib>:"Signals (Read).vi"("error in"=w770, "Mercury Reference In"=w773) -> ("error out"=w781:errorcluster, "Current"=→"M3 Current":dbl, "Mercury Reference Out"=w779:T36)  [unwired: 1 in, 6 out]
        n313 = call-poly <instrlib>:"Signals (Read).vi"("error in"=w781, "Mercury Reference In"=w779) -> ("error out"=w768:errorcluster, "Voltage"=→"M3 Voltage":dbl)  [unwired: 1 in, 7 out]
        n314 = call <vilib>:"Add State(s) to Queue__JKI_lib_State_Machine.vi"("State(s) in (\"\")"=w797) -> ("States Out"=w798:string)  [unwired: 14 in]
      }
      frame "Mercury: IPS: Idle - 2" {
        w804 = enum16{"write", "read"}."write" ("Function")
        # "set all of these things"
        n315 = Unbundle By Name(w812) -> ("Mercury IPS Ref"=w824:T36)
        n316 = local read "IPS Devices"() -> (w849:string[])
        n317 = Index Array(array=w849, index=0) -> (element=w848:string)
        n318 = call-poly <instrlib>:"Open.vi"("error in (no error)"=w845, "Device Identifier"=w848, "Mercury Reference In"=w824) -> ("error out"=w851:errorcluster, "Mercury Reference Out"=w852:T36)  [unwired: 7 out]
        n319 = call-poly <instrlib>:"Signals (Read).vi"("error in"=w851, "Mercury Reference In"=w852) -> ("error out"=w853:errorcluster, "Level"=w836:dbl, "Mercury Reference Out"=w854:T36)  [unwired: 1 in, 6 out]
        "He LVL Chart" <- w836
        n320 = Greater?(x=w836, y=20.0) -> (0:w843:bool)
        n321 = Greater?(x=w836, y=50.0) -> (0:w844:bool)
        n322 = call-poly <instrlib>:"Signals (Read).vi"("error in"=w853, "Mercury Reference In"=w854) -> ("error out"=w802:errorcluster, "Level"=w835:dbl)  [unwired: 1 in, 7 out]
        "N2 LVL Chart" <- w835
        n323 = case shown="False" w843 {
          tunnel: [w862 u32 6618880] -> w833
          tunnel: w844 -> [w863 _]
          frame False {
            n324 = case shown="False" w863 {
              tunnel: [u32 16711680 u32 16776704] -> w862
              frame False {
              }
              frame True {
              }
            }
          }
          frame True {
          }
        }
        n325 = local write "He LEVEL"(w836) -> ()
        n326 = property on="He LVL Chart" class="Slide (strict)"("Fill Color"=w833) -> ()  [unwired: 2 in, 2 out]
        n327 = property on="He LEVEL" class="DigNum (strict)"("NumText.TextColor"=w833) -> ()  [unwired: 2 in, 2 out]
        n328 = local write "N2 LEVEL"(w835) -> ()
        n329 = local read "Target Field Rate (T/min)"() -> (w829:dbl)
        n330 = local read "Power Supply Field (T)"() -> (w827:dbl)
        n331 = Greater?(x=w835, y=20.0) -> (0:w838:bool)
        n332 = Greater?(x=w835, y=50.0) -> (0:w837:bool)
        n333 = local read "Magnet Field (T)"() -> (w826:dbl)
        n334 = local read "Target Field (T)"() -> (w828:dbl)
        n335 = local read "Current (A)"() -> (w831:dbl)
        n336 = local read "Voltage (V)"() -> (w830:dbl)
        n337 = local read "SWITCH HEATER"() -> (w813:bool)
        n338 = local read "PSU Act Stat"() -> (w805:string)
        n339 = case shown="True" w838 {
          tunnel: [w857 u32 6618880] -> w834
          tunnel: w837 -> [w858 _]
          frame False {
            n340 = case shown="False" w858 {
              tunnel: [u32 16711680 u32 16776704] -> w857
              frame False {
              }
              frame True {
              }
            }
          }
          frame True {
          }
        }
        n341 = local read "Magnet Temperature"() -> (w822:dbl)
        n342 = property on="N2 LVL Chart" class="Slide (strict)"("Fill Color"=w834) -> ()  [unwired: 2 in, 2 out]
        n343 = property on="N2 LEVEL" class="DigNum (strict)"("NumText.TextColor"=w834) -> ()  [unwired: 2 in, 2 out]
        n344 = Bundle By Name(cluster=T29 {"Magnet Field"=0.0, "PS Field"=0.0, "Target Field"=0.0, "Target Field Rate"=0.0, "Voltage"=0.0, "Current"=0.0, "Switch"=FALSE, "Mercury State"=""} ("Status"), "Magnet Field"=w826, "PS Field"=w827, "Target Field"=w828, "Target Field Rate"=w829, "Voltage"=w830, "Current"=w831, "Switch"=w813, "Mercury State"=w805) -> (w810:T29)
        n345 = local read "Magnet Resistance"() -> (w823:dbl)
        n346 = Select(t="ON", s=w813, f="OFF") -> (s? t:f=w803:string)
        n347 = local read "M1 Current"() -> (w821:dbl)
        n348 = local read "M1 Voltage"() -> (w820:dbl)
        n349 = local read "M2 Current"() -> (w819:dbl)
        n350 = local read "M2 Voltage"() -> (w818:dbl)
        n351 = local read "M3 Current"() -> (w817:dbl)
        n352 = local read "M3 Voltage"() -> (w816:dbl)
        n353 = call "FGV_PSP - Mercury Status.vi"("error in"=w802, "Function"=w804, "Status"=w810) -> ("error out"=w809:errorcluster)  [unwired: 3 in, 1 out]
        n354 = Bundle(cluster=T30 {"Magnet Field"=0.0, "PS Field"=0.0, "Target Field"=0.0, "Target Field Rate"=0.0, "Voltage"=0.0, "Current"=0.0}, "Magnet Field"=w826, "PS Field"=w827, "Target Field"=w828, "Target Field Rate"=w829, "Voltage"=w830, "Current"=w831) -> (w832:T30)
        n355 = call "FGV_PSP - Mercury Action Status.vi"("error in"=w809, "Function"=w804, "Mercury Status"=w805) -> ("error out"=w808:errorcluster)  [unwired: 3 in, 1 out]
        n356 = Cluster To Array(cluster=w832) -> (array=w807:dbl[])
        n357 = Build Array(w821, w820, w819, w818, w817, w816) -> (w806:dbl[])
        n358 = Build Array (concatenate)(w807, w835, w836, w822, w823, w806) -> (w847:dbl[])
        n359 = Build Array(w805, w803) -> (w846:string[])
        n360 = call "1820_IPS_to_DSC.vi"("str"=w846, "dbl"=w847) -> ()  [unwired: 2 in]
        n361 = call <vilib>:"Add State(s) to Queue__JKI_lib_State_Machine.vi"("State(s) in (\"\")"=w855) -> ("States Out"=w856:string)  [unwired: 14 in]
      }
      frame "Mercury: IPS: Idle - 3" {
        n362 = call "Oxford_MNK_Omega_Sign.vi"("error in (no error)"=w868) -> ("error out"=w867:errorcluster)  [unwired: 10 in]
        n363 = call <vilib>:"Add State(s) to Queue__JKI_lib_State_Machine.vi"("State(s) in (\"\")"=w870) -> ("States Out"=w871:string)  [unwired: 14 in]
      }
      frame "Mercury: ITC: Idle" {
        n364 = Unbundle By Name(w893) -> ("Mercury ITC Ref"=w877:T36)
        n365 = local read "ITC Devices"() -> (w892:string[])
        n366 = Index Array(array=w892, index=1) -> (element=w890:string)
        n367 = call-poly <instrlib>:"Open.vi"("error in (no error)"=w872, "Device Identifier"=w890, "Mercury Reference In"=w877) -> ("error out"=w889:errorcluster, "Mercury Reference Out"=w888:T36)  [unwired: 7 out]
        n368 = call-poly <instrlib>:"Configuration (Read).vi"("error in"=w889, "Mercury Reference In"=w888) -> ("error out"=w886:errorcluster, "Device Details"=w887:T47)  [unwired: 1 in, 7 out]
        n369 = local read "ITC Devices"() -> (w884:string[])
        n370 = Unbundle By Name(w887) -> ("Pressure Signals.Pressure"=w876:string)
        n371 = Index Array(array=w884, index=0) -> (element=w883:string)
        n372 = Fract/Exp String To Number(string=w876) -> (number=w875:dbl)  [unwired: 3 in, 1 out]
        "LPF Pressure" <- w875
        n373 = call-poly <instrlib>:"Open.vi"("error in (no error)"=w886, "Device Identifier"=w883, "Mercury Reference In"=w877) -> ("error out"=w882:errorcluster, "Mercury Reference Out"=w881:T36)  [unwired: 7 out]
        n374 = local read "LPF Temperature"() -> (w874:dbl)
        n375 = local read "LPF Resistance"() -> (w873:dbl)
        n376 = call-poly <instrlib>:"Signals (Read).vi"("error in"=w882, "Mercury Reference In"=w881) -> ("error out"=w878:errorcluster, "% Open"=w879:dbl)  [unwired: 1 in, 7 out]
        "LPF Needle Valve (%)" <- w879
        n377 = Build Array(w874, w875, w879, w873) -> (w880:dbl[])
        n378 = call "1820_ITC_to_DSC.vi"("dbl"=w880) -> ()  [unwired: 3 in]
        n379 = call <vilib>:"Add State(s) to Queue__JKI_lib_State_Machine.vi"("State(s) in (\"\")"=w894) -> ("States Out"=w895:string)  [unwired: 14 in]
      }
      frame "Mercury: Empty" {
        n380 = call <vilib>:"Add State(s) to Queue__JKI_lib_State_Machine.vi"("State(s) in (\"\")"=w898) -> ("States Out"=w899:string)  [unwired: 14 in]
      }
      frame "---------- Mercury: Action ----------" {
        n381 = call <vilib>:"Add State(s) to Queue__JKI_lib_State_Machine.vi"("State(s) in (\"\")"=w903) -> ("States Out"=w902:string)  [unwired: 14 in]
      }
      frame "Mercury: Remote" {
        w918 = "\n"
        w911 = enum16{"write", "read"}."read" ("Function")
        n382 = call "FGV_PSP - Mercury Remote.vi"("error in"=w941, "Function"=enum16{"write", "read"}."write", "Remote"=TRUE ("Mercury FGV.Remote")) -> ("error out"=w940:errorcluster)  [unwired: 3 in, 1 out]
        n383 = call "FGV_PSP - Mercury Actions.vi"("error in"=w940, "Function"=w911) -> ("error out"=w916:errorcluster, "Actions"=w917:T31)  [unwired: 4 in]
        n384 = call "FGV_PSP - Mercury Targets.vi"("error in"=w916, "Function"=w911) -> ("error out"=w912:errorcluster, "Targets"=w915:T53)  [unwired: 4 in]
        n385 = Unbundle By Name(w915) -> ("Target Field (T)"=w914:dbl, "Target Field Rate (T/min)"=w913:dbl)
        n386 = Unbundle By Name(w917) -> ("Hold"=w910:bool, "Clamp"=w905:bool, "To Set"=w906:bool, "To Zero"=w907:bool, "PS Heat"=w908:bool, "Lambda"=w904:bool, "Send to IPS"=w909:bool)
        n387 = local read "Send to IPS"() -> (w932:bool)
        n388 = local read "Lambda"() -> (w931:bool)
        n389 = local read "To Zero"() -> (w929:bool)
        n390 = local read "PS Heat"() -> (w930:bool)
        n391 = local read "Clamp"() -> (w927:bool)
        n392 = local read "To Set"() -> (w928:bool)
        n393 = local read "Hold"() -> (w926:bool)
        n394 = local write "Send to IPS"(w909) -> ()
        n395 = local write "Lambda"(w904) -> ()
        n396 = local write "To Zero"(w907) -> ()
        n397 = local write "PS Heat"(w908) -> ()
        n398 = local write "Clamp"(w905) -> ()
        n399 = Not Equal?(x=w926, y=w910) -> (x != y?=w939:bool)
        n400 = Not Equal?(x=w927, y=w905) -> (x != y?=w938:bool)
        n401 = Not Equal?(x=w928, y=w906) -> (x != y?=w937:bool)
        n402 = local write "To Set"(w906) -> ()
        n403 = Not Equal?(x=w929, y=w907) -> (x != y?=w936:bool)
        n404 = Not Equal?(x=w930, y=w908) -> (x != y?=w935:bool)
        n405 = Not Equal?(x=w931, y=w904) -> (x != y?=w934:bool)
        n406 = Not Equal?(x=w932, y=w909) -> (x != y?=w933:bool)
        n407 = local write "Hold"(w910) -> ()
        n408 = local write "Target Field (T)"(w914) -> ()
        n409 = local write "Target Rate (T/min)"(w913) -> ()
        n410 = case shown="True" w939 {
          tunnel: ["" ("State(s) in Front (\"\")") "Mercury: Hold" ("State(s) in Front (\"\")")] -> w925
          frame False {
          }
          frame True {
          }
        }
        n411 = case shown="True" w937 {
          tunnel: ["" ("State(s) in Front (\"\")") "Mercury: To Set" ("State(s) in Front (\"\")")] -> w923
          frame False {
          }
          frame True {
          }
        }
        n412 = case shown="True" w935 {
          tunnel: ["" ("State(s) in Front (\"\")") "Mercury: PS Heat" ("State(s) in Front (\"\")")] -> w921
          frame False {
          }
          frame True {
          }
        }
        n413 = case shown="True" w934 {
          tunnel: ["" ("State(s) in Front (\"\")") "Mercury: Lambda" ("State(s) in Front (\"\")")] -> w920
          frame False {
          }
          frame True {
          }
        }
        n414 = case shown="True" w933 {
          tunnel: ["" ("State(s) in Front (\"\")") "Mercury: Send To IPS" ("State(s) in Front (\"\")")] -> w919
          frame False {
          }
          frame True {
          }
        }
        n415 = case shown="True" w938 {
          tunnel: ["" ("State(s) in Front (\"\")") "Mercury: Clamp" ("State(s) in Front (\"\")")] -> w924
          frame False {
          }
          frame True {
          }
        }
        n416 = case shown="True" w936 {
          tunnel: ["" ("State(s) in Front (\"\")") "Mercury: To Zero" ("State(s) in Front (\"\")")] -> w922
          frame False {
          }
          frame True {
          }
        }
        n417 = Concatenate Strings(w925, w918, w924, w918, w923, w918, w922, w918, w921, w918, w920, w918, w919, w918) -> (w945:string)
        n418 = call <vilib>:"Add State(s) to Queue__JKI_lib_State_Machine.vi"("State(s) in Front (\"\")"=w945, "State(s) in (\"\")"=w946) -> ("States Out"=w947:string)  [unwired: 13 in]
      }
      frame "Mercury: Hold" {
        w963 = FALSE ("Hold")
        n419 = Unbundle By Name(w968) -> ("Mercury IPS Ref"=w976:T36)
        n420 = local read "Device Identifier"() -> (w977:T24)
        n421 = call-poly <instrlib>:"Open.vi"("error in (no error)"=w974, "Device Identifier"=w977, "Mercury Reference In"=w976) -> ("error out"=w978:errorcluster, "Mercury Reference Out"=w975:T36)  [unwired: 7 out]
        n422 = call-poly <instrlib>:"Signals (Set).vi"("error in"=w978, "PSU Act Stat"=T32 "HOLD", "Mercury Reference In"=w975) -> ("error out"=w971:errorcluster, "Response"=w969:T35)  [unwired: 1 in, 6 out]
        n423 = call "IPSReplytoDSC.vi"("error in (no error)"=w971, "Response"=w969) -> ("error out"=w964:errorcluster)  [unwired: 9 in]
        n424 = call "MercuryStateHistory.vi"("initialize?"=FALSE, "Current State in"=w969) -> ("delimited string"=w972:string)  [unwired: 8 in, 1 out]
        n425 = local write "Magnet Status 2"(w972) -> ()
        n426 = local write "Hold"(w963) -> ()
        n427 = Bundle By Name(cluster=T31 {"Hold"=FALSE, "Clamp"=FALSE, "To Set"=FALSE, "To Zero"=FALSE, "Send to IPS"=FALSE, "PS Heat"=FALSE, "Lambda"=FALSE} ("Actions"), "Hold"=w963) -> (w966:T31)
        n428 = call "FGV_PSP - Mercury Actions.vi"("error in"=w964, "Function"=enum16{"write", "read"}."write", "Actions"=w966) -> ("error out"=w962:errorcluster)  [unwired: 3 in, 1 out]
        n429 = call <vilib>:"Add State(s) to Queue__JKI_lib_State_Machine.vi"("State(s) in (\"\")"=w979) -> ("States Out"=w980:string)  [unwired: 14 in]
      }
      frame "Mercury: Clamp" {
        w981 = FALSE
        n430 = Unbundle By Name(w987) -> ("Mercury IPS Ref"=w994:T36)
        n431 = local read "Device Identifier"() -> (w997:T24)
        n432 = call-poly <instrlib>:"Open.vi"("error in (no error)"=w993, "Device Identifier"=w997, "Mercury Reference In"=w994) -> ("error out"=w996:errorcluster, "Mercury Reference Out"=w995:T36)  [unwired: 7 out]
        n433 = call-poly <instrlib>:"Signals (Set).vi"("error in"=w996, "PSU Act Stat"=T32 "CLMP", "Mercury Reference In"=w995) -> ("error out"=w991:errorcluster, "Response"=w988:T35)  [unwired: 1 in, 6 out]
        n434 = call "IPSReplytoDSC.vi"("error in (no error)"=w991, "Response"=w988) -> ("error out"=w983:errorcluster)  [unwired: 9 in]
        n435 = call "MercuryStateHistory.vi"("initialize?"=FALSE, "Current State in"=w988) -> ("delimited string"=w989:string)  [unwired: 8 in, 1 out]
        n436 = local write "Magnet Status 2"(w989) -> ()
        n437 = local write "Clamp"(w981) -> ()
        n438 = Bundle By Name(cluster=T31 {"Hold"=FALSE, "Clamp"=FALSE, "To Set"=FALSE, "To Zero"=FALSE, "Send to IPS"=FALSE, "PS Heat"=FALSE, "Lambda"=FALSE} ("Actions"), "Clamp"=w981) -> (w985:T31)
        n439 = call "FGV_PSP - Mercury Actions.vi"("error in"=w983, "Function"=enum16{"write", "read"}."write", "Actions"=w985) -> ("error out"=w982:errorcluster)  [unwired: 3 in, 1 out]
        n440 = call <vilib>:"Add State(s) to Queue__JKI_lib_State_Machine.vi"("State(s) in (\"\")"=w998) -> ("States Out"=w999:string)  [unwired: 14 in]
      }
      frame "Mercury: To Set" {
        w1002 = FALSE
        n441 = Unbundle By Name(w1006) -> ("Mercury IPS Ref"=w1014:T36)
        n442 = local read "Device Identifier"() -> (w1013:T24)
        n443 = call-poly <instrlib>:"Open.vi"("error in (no error)"=w1012, "Device Identifier"=w1013, "Mercury Reference In"=w1014) -> ("error out"=w1015:errorcluster, "Mercury Reference Out"=w1016:T36)  [unwired: 7 out]
        n444 = call-poly <instrlib>:"Signals (Set).vi"("error in"=w1015, "PSU Act Stat"=T32 "RTOS", "Mercury Reference In"=w1016) -> ("error out"=w1009:errorcluster, "Response"=w1008:T35)  [unwired: 1 in, 6 out]
        n445 = call "IPSReplytoDSC.vi"("error in (no error)"=w1009, "Response"=w1008) -> ("error out"=w1001:errorcluster)  [unwired: 9 in]
        n446 = call "MercuryStateHistory.vi"("initialize?"=FALSE, "Current State in"=w1008) -> ("delimited string"=w1010:string)  [unwired: 8 in, 1 out]
        n447 = local write "Magnet Status 2"(w1010) -> ()
        n448 = local write "To Set"(w1002) -> ()
        n449 = Bundle By Name(cluster=T31 {"Hold"=FALSE, "Clamp"=FALSE, "To Set"=FALSE, "To Zero"=FALSE, "Send to IPS"=FALSE, "PS Heat"=FALSE, "Lambda"=FALSE} ("Actions"), "To Set"=w1002) -> (w1004:T31)
        n450 = call "FGV_PSP - Mercury Actions.vi"("error in"=w1001, "Function"=enum16{"write", "read"}."write", "Actions"=w1004) -> ("error out"=w1000:errorcluster)  [unwired: 3 in, 1 out]
        n451 = call <vilib>:"Add State(s) to Queue__JKI_lib_State_Machine.vi"("State(s) in (\"\")"=w1017) -> ("States Out"=w1018:string)  [unwired: 14 in]
      }
      frame "Mercury: To Zero" {
        w1021 = FALSE
        n452 = Unbundle By Name(w1025) -> ("Mercury IPS Ref"=w1033:T36)
        n453 = local read "Device Identifier"() -> (w1032:T24)
        n454 = call-poly <instrlib>:"Open.vi"("error in (no error)"=w1031, "Device Identifier"=w1032, "Mercury Reference In"=w1033) -> ("error out"=w1034:errorcluster, "Mercury Reference Out"=w1035:T36)  [unwired: 7 out]
        n455 = call-poly <instrlib>:"Signals (Set).vi"("error in"=w1034, "PSU Act Stat"=T32 "RTOZ", "Mercury Reference In"=w1035) -> ("error out"=w1028:errorcluster, "Response"=w1026:T35)  [unwired: 1 in, 6 out]
        n456 = call "IPSReplytoDSC.vi"("error in (no error)"=w1028, "Response"=w1026) -> ("error out"=w1020:errorcluster)  [unwired: 9 in]
        n457 = call "MercuryStateHistory.vi"("initialize?"=FALSE, "Current State in"=w1026) -> ("delimited string"=w1029:string)  [unwired: 8 in, 1 out]
        n458 = local write "Magnet Status 2"(w1029) -> ()
        n459 = local write "To Zero"(w1021) -> ()
        n460 = Bundle By Name(cluster=T31 {"Hold"=FALSE, "Clamp"=FALSE, "To Set"=FALSE, "To Zero"=FALSE, "Send to IPS"=FALSE, "PS Heat"=FALSE, "Lambda"=FALSE} ("Actions"), "To Zero"=w1021) -> (w1023:T31)
        n461 = call "FGV_PSP - Mercury Actions.vi"("error in"=w1020, "Function"=enum16{"write", "read"}."write", "Actions"=w1023) -> ("error out"=w1019:errorcluster)  [unwired: 3 in, 1 out]
        n462 = call <vilib>:"Add State(s) to Queue__JKI_lib_State_Machine.vi"("State(s) in (\"\")"=w1036) -> ("States Out"=w1037:string)  [unwired: 14 in]
      }
      frame "Mercury: PS Heat" {
        # "set switch action to F because we\nalready changed it"
        # "set the status of the switch\nT = ON\nF = OFF"
        n463 = local read "Device Identifier"() -> (w1048:T24)
        n464 = Unbundle By Name(w1043) -> ("Mercury IPS Ref"=w1049:T36)
        n465 = call-poly <instrlib>:"Open.vi"("error in (no error)"=w1045, "Device Identifier"=w1048, "Mercury Reference In"=w1049) -> ("error out"=w1046:errorcluster, "Mercury Reference Out"=w1047:T36)  [unwired: 7 out]
        n466 = call-poly <instrlib>:"Signals (Read).vi"("error in"=w1046, "Mercury Reference In"=w1047) -> ("error out"=w1051:errorcluster, "Current"=w1040:dbl, "Mercury Reference Out"=w1050:T36)  [unwired: 1 in, 6 out]
        n467 = call-poly <instrlib>:"Signals (Read).vi"("error in"=w1051, "Mercury Reference In"=w1050) -> ("error out"=w1052:errorcluster, "Persistant Current"=w1039:dbl, "Mercury Reference Out"=w1053:T36)  [unwired: 1 in, 6 out]
        n468 = Subtract(x=w1039, y=w1040) -> (x-y=w1054:dbl)
        n469 = Absolute Value(x=w1054) -> (abs(x)=w1055:dbl)
        n470 = Less?(x=w1055, y=0.1) -> (x < y?=w1057:bool)
        n471 = case shown="False" w1057 {
          selector: w1057 -> [_ w1062]
          tunnel: [w1061 w1062] -> w1038
          frame False {
            n472 = Two Button Dialog(message="The magnet current is more\nthan 0.1A different to the\nPSU output current.  It is not\nadvisable to switch on the\nswitch heater unless these\ncurrents are equal!") -> (T button?=w1061:bool)  [unwired: 2 out]
          }
          frame True {
          }
        }
        n473 = local read "PS Heat"() -> (w1042:bool)
        n474 = Or(x=w1038, y=w1042) -> (x .or. y?=w1041:bool)
        n475 = case shown="True" w1041 {
          tunnel: w1053 -> [_ w1092]
          tunnel: w1052 -> [w1063 w1091]
          tunnel: [w1063 w1078] -> w1044
          frame False {
          }
          frame True {
            w1064 = FALSE ("PS Heat")
            n476 = Get Date/Time In Seconds() -> (seconds since 1Jan1904=→"PS ON/OFF":timestamp)
            n477 = call-poly <instrlib>:"Signals (Read).vi"("error in"=w1091, "Mercury Reference In"=w1092) -> ("error out"=w1093:errorcluster, "Switch Heater Status"=w1074:string, "Mercury Reference Out"=w1075:T36)  [unwired: 1 in, 6 out]
            n478 = Equal?(x=w1074, y="ON") -> (x = y?=w1072:bool)
            n479 = call <userlib>:"Wait (ms)__ogtk.vi"("error in (no error)"=w1093, "milliseconds to wait"=u32 100 ("millisecond multiple")) -> ("error out"=w1090:errorcluster)  [unwired: 8 in, 1 out]
            n480 = Select(t=T33 "OFF" ("Set Switch Heater"), s=w1072, f=T33 "ON" ("Set Switch Heater")) -> (s? t:f=w1067:T33)
            n481 = call-poly <instrlib>:"Signals (Set).vi"("error in"=w1090, "Set Switch Heater"=w1067, "Mercury Reference In"=w1075) -> ("error out"=w1084:errorcluster, "Response"=w1082:T35, "Mercury Reference Out"=w1071:T36)  [unwired: 1 in, 5 out]
            n482 = call "MercuryStateHistory.vi"("initialize?"=FALSE, "Current State in"=w1082) -> ("delimited string"=w1086:string)  [unwired: 8 in, 1 out]
            n483 = local write "Magnet Status 2"(w1086) -> ()
            n484 = call "IPSReplytoDSC.vi"("error in (no error)"=w1084, "Response"=w1082) -> ("error out"=w1081:errorcluster)  [unwired: 9 in]
            n485 = while {
              tunnel: [w1101] -> w1076
              tunnel: w1081 -> [w1099]
              tunnel: w1067 -> [w1097]
              tunnel: w1071 -> [w1095]
              tunnel: [w1094] -> w1066
              stop <- w1096 stop-if-true
              # "wait here while setting"
              n486 = call-poly <instrlib>:"Signals (Read).vi"("error in"=w1099, "Mercury Reference In"=w1095) -> ("error out"=w1101:errorcluster, "Switch Heater Status"=w1098:string)  [unwired: 1 in, 7 out]
              n487 = Equal?(x=w1098, y=w1097) -> (x = y?=w1096:bool)
              n488 = Equal?(x=w1098, y="ON") -> (x = y?=w1094:bool)
            }
            n489 = Bundle By Name(cluster=T29 {"Magnet Field"=0.0, "PS Field"=0.0, "Target Field"=0.0, "Target Field Rate"=0.0, "Voltage"=0.0, "Current"=0.0, "Switch"=FALSE, "Mercury State"=""} ("Status"), "Switch"=w1066) -> (w1069:T29)
            n490 = call "FGV_PSP - Mercury Status.vi"("error in"=w1076, "Function"=enum16{"write", "read"}."write", "Status"=w1069) -> ("error out"=w1077:errorcluster)  [unwired: 3 in, 1 out]
            n491 = local write "PS Heat"(w1064) -> ()
            n492 = Bundle By Name(cluster=T31 {"Hold"=FALSE, "Clamp"=FALSE, "To Set"=FALSE, "To Zero"=FALSE, "Send to IPS"=FALSE, "PS Heat"=FALSE, "Lambda"=FALSE} ("Actions"), "PS Heat"=w1064) -> (w1079:T31)
            n493 = call "FGV_PSP - Mercury Actions.vi"("error in"=w1077, "Function"=enum16{"write", "read"}."write", "Actions"=w1079) -> ("error out"=w1078:errorcluster)  [unwired: 3 in, 1 out]
          }
        }
        n494 = call <vilib>:"Add State(s) to Queue__JKI_lib_State_Machine.vi"("State(s) in (\"\")"=w1058) -> ("States Out"=w1059:string)  [unwired: 14 in]
      }
      frame "Mercury: Send To IPS" {
        w1103 = FALSE
        n495 = local read "Device Identifier"() -> (w1124:T24)
        n496 = Unbundle By Name(w1111) -> ("Mercury IPS Ref"=w1123:T36)
        n497 = call-poly <instrlib>:"Open.vi"("error in (no error)"=w1121, "Device Identifier"=w1124, "Mercury Reference In"=w1123) -> ("error out"=w1125:errorcluster, "Mercury Reference Out"=w1122:T36)  [unwired: 7 out]
        n498 = call-poly <instrlib>:"Signals (Set).vi"("error in"=w1125, "Target Field Rate"="Target Rate (T/min)", "Mercury Reference In"=w1122) -> ("error out"=w1119:errorcluster, "Response"=w1117:T35, "Mercury Reference Out"=w1110:T36)  [unwired: 2 in, 4 out]
        n499 = call "MercuryStateHistory.vi"("initialize?"=FALSE, "Current State in"=w1117) -> ("delimited string"=w1113:string)  [unwired: 8 in, 1 out]
        n500 = call "IPSReplytoDSC.vi"("error in (no error)"=w1119, "Response"=w1117) -> ("error out"=w1118:errorcluster)  [unwired: 9 in]
        n501 = local write "Magnet Status 2"(w1113) -> ()
        n502 = call-poly <instrlib>:"Signals (Set).vi"("error in"=w1118, "Target Field"="Target Field (T)", "Mercury Reference In"=w1110) -> ("error out"=w1120:errorcluster, "Response"=w1112:T35)  [unwired: 2 in, 5 out]
        n503 = local write "Send to IPS"(w1103) -> ()
        n504 = call "IPSReplytoDSC.vi"("error in (no error)"=w1120, "Response"=w1112) -> ("error out"=w1104:errorcluster)  [unwired: 9 in]
        n505 = call "MercuryStateHistory.vi"("initialize?"=FALSE, "Current State in"=w1112) -> ("delimited string"=w1114:string)  [unwired: 8 in, 1 out]
        n506 = local write "Magnet Status 2"(w1114) -> ()
        n507 = Bundle By Name(cluster=T31 {"Hold"=FALSE, "Clamp"=FALSE, "To Set"=FALSE, "To Zero"=FALSE, "Send to IPS"=FALSE, "PS Heat"=FALSE, "Lambda"=FALSE} ("Actions"), "Send to IPS"=w1103) -> (w1106:T31)
        n508 = call "FGV_PSP - Mercury Actions.vi"("error in"=w1104, "Function"=enum16{"write", "read"}."write", "Actions"=w1106) -> ("error out"=w1102:errorcluster)  [unwired: 3 in, 1 out]
        n509 = call <vilib>:"Add State(s) to Queue__JKI_lib_State_Machine.vi"("State(s) in (\"\")"=w1126) -> ("States Out"=w1127:string)  [unwired: 14 in]
      }
      frame "Mercury: Lambda" {
        # "AUX\nPRES\nHTR\nTEMP"
        n510 = Unbundle By Name(w1134) -> ("Mercury ITC Ref"=w1146:T36)
        n511 = local read "Lambda"() -> (w1129:bool)
        n512 = call-poly <instrlib>:"Open.vi"("error in (no error)"=w1135, "Device Identifier"="lambda:LPC", "Mercury Reference In"=w1146) -> ("error out"=w1143:errorcluster, "Mercury Reference Out"=w1142:T36)  [unwired: 7 out]
        n513 = Select(t="ON" ("Sweep Mode"), s=w1129, f="OFF" ("Sweep Mode")) -> (s? t:f=w1141:string)
        n514 = case shown="False" w1129 {
          frame False {
            n515 = disable-structure shown="Disabled" {
              frame Disabled {
                n516 = property on="Close Needle Valve" class="Bool (strict)"("Val(Sgnl)"=TRUE ("Value (Signaling)")) -> ()  [unwired: 2 in, 2 out]
              }
              frame Enabled {
              }
            }
          }
          frame True {
          }
        }
        n517 = case shown="False" w1129 {
          frame False {
            n518 = local write "LPF ON"(timestamp(0 s since 1904-01-01) ("LPF ON")) -> ()
          }
          frame True {
            n519 = Get Date/Time In Seconds() -> (seconds since 1Jan1904=w1151:timestamp)
            n520 = local write "LPF ON"(w1151) -> ()
          }
        }
        n521 = call-poly <instrlib>:"Configuration (Set).vi"("error in"=w1143, "Lambda Auto"=w1141, "Mercury Reference In"=w1142) -> ("error out"=w1139:errorcluster, "Response"=w1138:T35)  [unwired: 5 in, 2 out]
        n522 = call "ITCReplytoDSC.vi"("error in (no error)"=w1139, "Response"=w1138) -> ("error out"=w1130:errorcluster)  [unwired: 9 in]
        n523 = call "MercuryStateHistory.vi"("initialize?"=FALSE, "Current State in"=w1138) -> ("delimited string"=w1136:string)  [unwired: 8 in, 1 out]
        n524 = local write "Magnet Status 2"(w1136) -> ()
        n525 = Bundle By Name(cluster=T31 {"Hold"=FALSE, "Clamp"=FALSE, "To Set"=FALSE, "To Zero"=FALSE, "Send to IPS"=FALSE, "PS Heat"=FALSE, "Lambda"=FALSE} ("Actions"), "Lambda"=w1129) -> (w1132:T31)
        n526 = call "FGV_PSP - Mercury Actions.vi"("error in"=w1130, "Function"=enum16{"write", "read"}."write", "Actions"=w1132) -> ("error out"=w1128:errorcluster)  [unwired: 3 in, 1 out]
        n527 = call <vilib>:"Add State(s) to Queue__JKI_lib_State_Machine.vi"("State(s) in (\"\")"=w1147) -> ("States Out"=w1148:string)  [unwired: 14 in]
      }
      frame "Mercury: Fast/Slow Fill" {
        n528 = local read "IPS Devices"() -> (w1166:string[])
        n529 = Unbundle By Name(w1152) -> ("Mercury IPS Ref"=w1168:T36)
        n530 = local read "Fast/Slow Fill"() -> (w1153:bool)
        n531 = Index Array(array=w1166, index=0) -> (element=w1161:string)
        n532 = call-poly <instrlib>:"Open.vi"("error in (no error)"=w1155, "Device Identifier"=w1161, "Mercury Reference In"=w1168) -> ("error out"=w1163:errorcluster, "Mercury Reference Out"=w1164:T36)  [unwired: 7 out]
        n533 = Select(t="OFF" ("Temperature setpoint"), s=w1153, f="ON" ("Temperature setpoint")) -> (s? t:f=w1165:string)
        n534 = call-poly <instrlib>:"Configuration (Set).vi"("ISOBUS address"=T34 -1, "error in"=w1163, "Delay"=w1165, "Mercury Reference In"=w1164) -> ("error out"=w1157:errorcluster, "Response"=w1156:T35)  [unwired: 4 in, 2 out]
        n535 = call "MercuryStateHistory.vi"("Current State in"=w1156) -> ("delimited string"=w1158:string)  [unwired: 9 in, 1 out]
        n536 = call "IPSReplytoDSC.vi"("error in (no error)"=w1157, "Response"=w1156) -> ("error out"=w1154:errorcluster)  [unwired: 9 in]
        n537 = local write "Magnet Status 2"(w1158) -> ()
        n538 = call <vilib>:"Add State(s) to Queue__JKI_lib_State_Machine.vi"("State(s) in (\"\")"=w1169) -> ("States Out"=w1170:string)  [unwired: 14 in]
      }
      frame "Mercury: Needle Valve" {
        n539 = Unbundle By Name(w1173) -> ("Mercury ITC Ref"=w1185:T36)
        n540 = Build Array("Close Needle Valve", "Open Needle Valve") -> (w1181:bool[])
        n541 = call-poly <instrlib>:"Open.vi"("error in (no error)"=w1171, "Device Identifier"="lambda:LPC", "Mercury Reference In"=w1185) -> ("error out"=w1180:errorcluster, "Mercury Reference Out"=w1179:T36)  [unwired: 7 out]
        n542 = Boolean Array To Number(Boolean array=w1181) -> (number=w1178:u32)
        n543 = case shown="0, Default" w1178 {
          tunnel: w1180 -> [w1190 w1194 w1203]
          tunnel: w1179 -> [_ w1195 w1202]
          tunnel: [w1190 w1193 w1201] -> w1175
          tunnel: [T35 "" ("Response") w1192 w1200] -> w1174
          tunnel: [FALSE ("Close Needle Valve") FALSE ("Close Needle Valve") FALSE ("Close Needle Valve")] -> w1177
          frame 0, Default {
          }
          frame 1 {
            n544 = call-poly <instrlib>:"Configuration (Set).vi"("ISOBUS address"=T34 -1, "error in"=w1194, "Percentage Open"=0.0, "Mercury Reference In"=w1195) -> ("error out"=w1193:errorcluster, "Response"=w1192:T35)  [unwired: 4 in, 2 out]
          }
          frame 2 {
            n545 = call-poly <instrlib>:"Configuration (Set).vi"("ISOBUS address"=T34 -1, "error in"=w1203, "Percentage Open"="Percentage Open", "Mercury Reference In"=w1202) -> ("error out"=w1201:errorcluster, "Response"=w1200:T35)  [unwired: 4 in, 2 out]
          }
        }
        n546 = local write "Close Needle Valve"(w1177) -> ()
        n547 = local write "Open Needle Valve"(w1177) -> ()
        n548 = call "ITCReplytoDSC.vi"("error in (no error)"=w1175, "Response"=w1174) -> ("error out"=w1172:errorcluster)  [unwired: 9 in]
        n549 = call "MercuryStateHistory.vi"("Current State in"=w1174) -> ("delimited string"=w1176:string)  [unwired: 9 in, 1 out]
        n550 = local write "Magnet Status 2"(w1176) -> ()
        n551 = call <vilib>:"Add State(s) to Queue__JKI_lib_State_Machine.vi"("State(s) in (\"\")"=w1186) -> ("States Out"=w1187:string)  [unwired: 14 in]
      }
    }
  }
  n552 = disable-structure shown="Disabled" {
    frame Disabled {
      (unwired) FALSE
      n553 = call-poly <instrlib>:"Configuration (Read).vi"() -> ()  [unwired: 3 in, 9 out]
      n554 = disable-structure shown="Disabled" {
        frame Disabled {
          n555 = property on="Fast/Slow Fill" class="Bool (strict)" props=["Val(Sgnl)"]() -> ()  [unwired: 3 in, 2 out]
        }
        frame Enabled {
        }
      }
      n556 = local read "PS Heat"() -> ()  [unwired: 1 in]
      n557 = local read "Lambda"() -> ()  [unwired: 1 in]
      n558 = call-poly <instrlib>:"Configuration (Set).vi"("Password"="abc123", "Mode"=T42 "ENG") -> ("error out"=w1211:errorcluster, "Mercury Reference Out"=w1208:T36, "error in"=w1210:errorcluster, "Mercury Reference In"=w1205:T36)  [unwired: 4 in, 2 out]
      n559 = call-poly <instrlib>:"Configuration (Set).vi"("error in"=w1211, "Swh Htr Current"=90.0, "Mercury Reference In"=w1208) -> ("error out"=w1212:errorcluster, "Mercury Reference Out"=w1213:T36)  [unwired: 5 in, 2 out]
      n560 = call-poly <instrlib>:"Configuration (Set).vi"("error in"=w1212, "Mode"=T42 "NORM", "Mercury Reference In"=w1213) -> ()  [unwired: 5 in, 4 out]
      n561 = call-poly <instrlib>:"Signals (Read).vi"() -> ()  [unwired: 3 in, 9 out]
    }
    frame Enabled {
    }
  }
